vi "transfer char run_subvi_8_24_12a_JW.vi"(0 "VISA session":refnum<visa-resource-name>="GPIB0::17::INSTR", 5 "Var1 sweep settings":T7={"start"=40.0, "stop"=-40.0, "step (linear only)"=-1.0, "sweep spacing (linear: 0)"=0, "sweep mode"=FALSE, "compliance (V)"=100.0, "compliance (A)"=0.001} {"compliance (A)" format="%^.2e"; "compliance (V)" format="%.2f"; "sweep spacing (linear: 0)" items=["linear", "log 10", "log 25", "log 50"]; "step (linear only)" format="%.2f"; "stop" format="%.2f"; "start" format="%.2f"}, 7 "Var2 step settings":T6={"compliance (A)"=0.001, "compliance (V)"=100.0, "start"=-2.0, "total points"=2, "step"=-38.0} {"step" format="%.2f"; "start" format="%.2f"; "compliance (V)" format="%.2f"; "compliance (A)" format="%^.2e"}, 9 "integration time":u32(slide) scale=0.0..2.0, 11 "Input Path":path, 13 "Sample Properties:":T4 {"Date Created" format="%<%x>T"}) -> (2 "Check Cluster":T2, 4 "Output":T3 {"Mobility-Lin" format="%#_4e"; "Mobility-Sat" format="%#_4e"}, 6 "Graph Cluster":T1, 15 "error?":errorcluster)   [LabVIEW 2012]
uses:
  <vilib>/Utility/file.llb/Write To Spreadsheet File (DBL).vi
panel:
  in  "Output Path":path
  in  "Temp (K)":dbl=0.001 format="%^.2e"
  in  "NumPts":dbl=5.0
  out "Numeric":dbl
  out "min r":dbl
  out "max r":dbl
  out "error? 2":errorcluster
  in  "MAXIMUM":ext format="%.2e"
  in  "MINIMUM":ext=-1e-05 format="%_2e"
  out "Gate Current Plot":cluster{"trace":dbl[], "trace":dbl[]}(graph)
  in  "Y1 axis":string="Id"
  in  "Y2 axis settings":T5 {"MAXIMUM" format="%.9f"; "MINIMUM" format="%.9f"}
  out "graphic display":cluster{"trace":dbl[], "trace":dbl[]}(graph)
  in  "wait time parameter":dbl=1.0
  in  "Value (Either V or A) 4":dbl
  in  "Value (Either V or A) 3":dbl
  in  "Value (Either V or A) 2":dbl
  in  "Value (V or A)":dbl
  in  "compliance (A)":dbl=0.001 format="%^.2e"
  in  "compliance (V)":dbl=100.0 format="%^.2e"
  in  "Iname":string="Is"
  in  "Vname":string="Vs"
  in  "Function":u16(ring)=4 items=["disabled", "Var1", "Var2", "Var1'", "Constant"]
  in  "Mode":u16(ring)=4 items=["V", "I", "VPulse", "IPulse", "Common"]
  in  "Iname 4":string="I4"
  in  "Vname 4":string="V4"
  in  "Function 4":u16(ring)=4 items=["disabled", "Var1", "Var2", "Var1'", "Constant"]
  in  "Mode 4":u16(ring) items=["V", "I", "VPulse", "IPulse", "Common"]
  in  "Iname 3":string="Ig"
  in  "Vname 3":string="Vg"
  in  "Function 3":u16(ring)=1 items=["disabled", "Var1", "Var2", "Var1'", "Constant"]
  in  "Mode 3":u16(ring) items=["V", "I", "VPulse", "IPulse", "Common"]
  in  "Iname 2":string="Id"
  in  "Vname 2":string="Vd"
  in  "Function 2":u16(ring)=2 items=["disabled", "Var1", "Var2", "Var1'", "Constant"]
  in  "Mode 2":u16(ring) items=["V", "I", "VPulse", "IPulse", "Common"]
  in  "reset":bool=TRUE
  # "SMU1"
  # "SMU2"
  # "SMU3"
  # "SMU4"
  # "Sample Properties:"
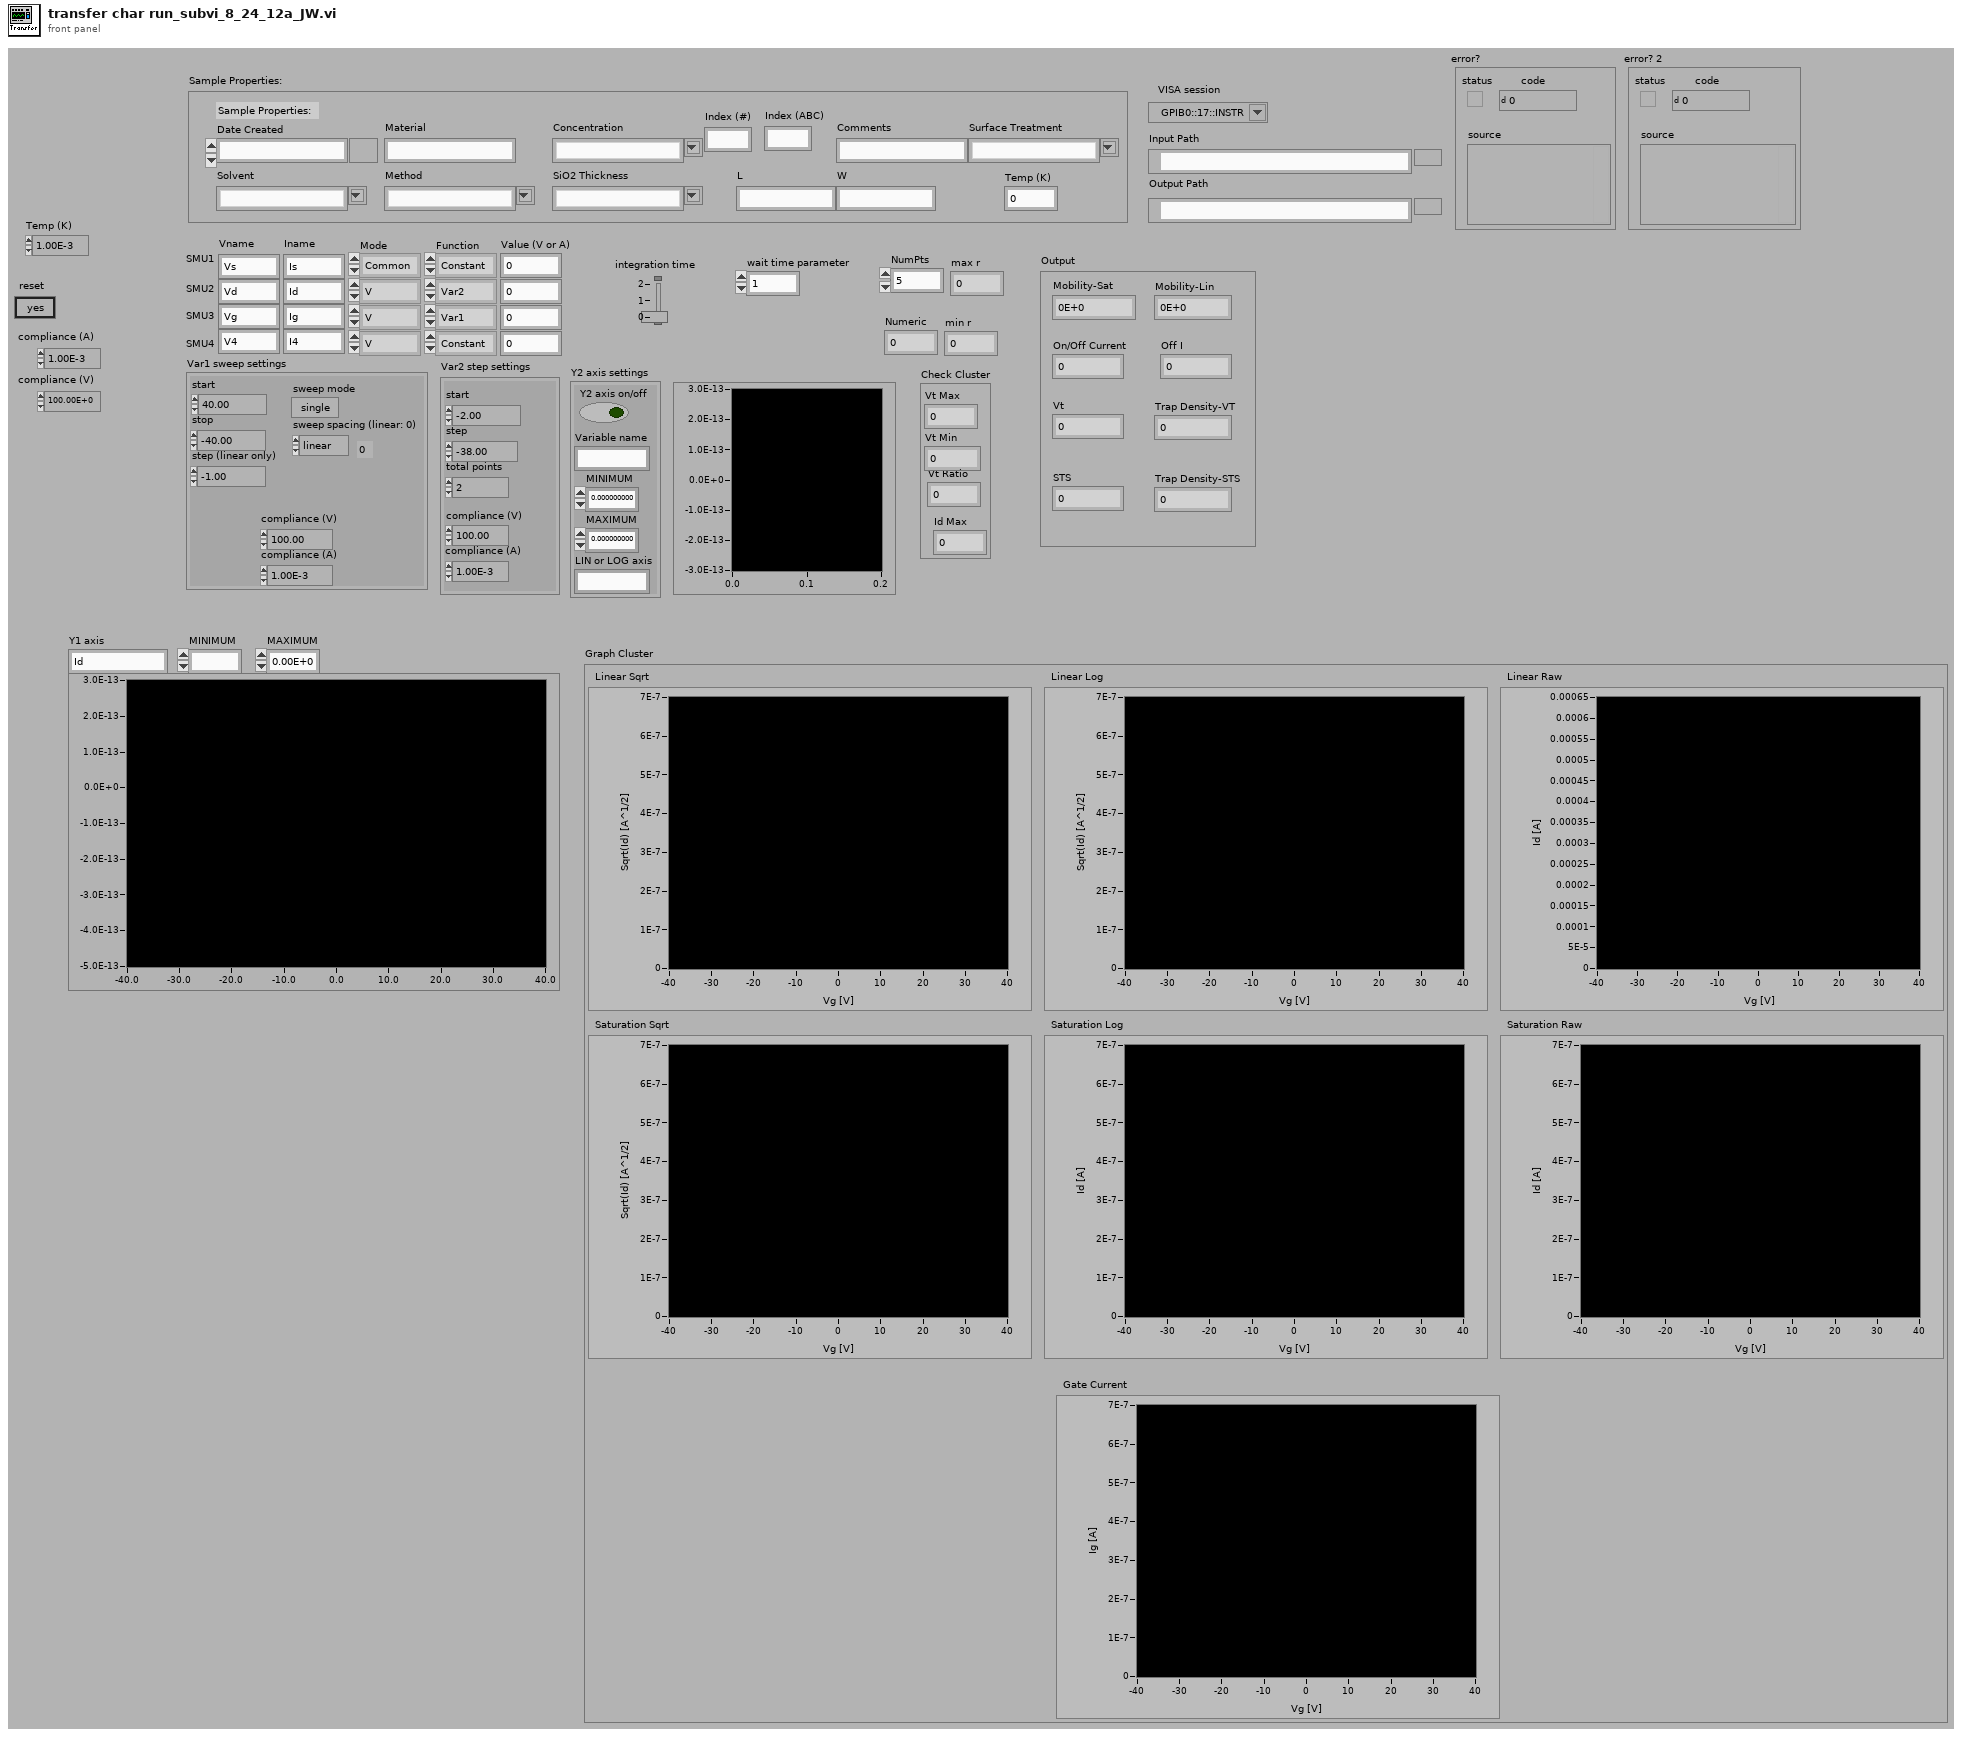
[diagram p1: front panel]
types:
  T1 = cluster{"Linear Sqrt":cluster{dbl[], "trace":dbl[]}[], "Linear Log":cluster{dbl[], "trace":dbl[]}[], "Linear Raw":cluster{dbl[], dbl[]}[], "Saturation Sqrt":cluster{dbl[], "trace":dbl[]}[], "Saturation Log":cluster{dbl[], "trace":dbl[]}[], "Saturation Raw":cluster{dbl[], "trace":dbl[]}[], "Gate Current":cluster{dbl[], "trace":dbl[]}[]}
  T2 = cluster{"Vt Max":i32, "Vt Min":i32, "Vt Ratio":i32, "Id Max":dbl}
  T3 = cluster{"Mobility-Sat":dbl, "Mobility-Lin":dbl, "On/Off Current":dbl, "Off I":dbl, "Vt":dbl, "STS":dbl, "Trap Density-VT":dbl, "Trap Density-STS":dbl}
  T4 = cluster{"Date Created":timestamp, "Material":string, "Solvent":string, "Concentration":string, "Method":string, "SiO2 Thickness":string, "Index (#)":string, "Index (ABC)":string, "L":string, "W":string, "Surface Treatment":string, "Comments":string, "Temp (K)":dbl}
  T5 = cluster{"Y2 axis on/off":bool, "MINIMUM":ext, "MAXIMUM":ext, "Variable name":string, "LIN or LOG axis":string}
  T6 = cluster{"compliance (A)":dbl, "compliance (V)":dbl, "start":dbl, "total points":u16, "step":dbl}
  T7 = cluster{"start":dbl, "stop":dbl, "step (linear only)":dbl, "sweep spacing (linear: 0)":u16, "sweep mode":bool, "compliance (V)":dbl, "compliance (A)":dbl}
  T8 = cluster{"Vt Max":dbl, "Vt Min":dbl, "Vt Ratio":dbl, "Id Max":dbl}
  T9 = cluster{"Mobility-Sat":dbl, "Mobility-Lin":dbl, "On/Off I-Sat":dbl, "Off I-Sat":dbl, "VT-Sat":dbl, "Sub Threshold Swing":dbl, "Trap Density-VT":dbl, "Trap Density (N)":dbl}
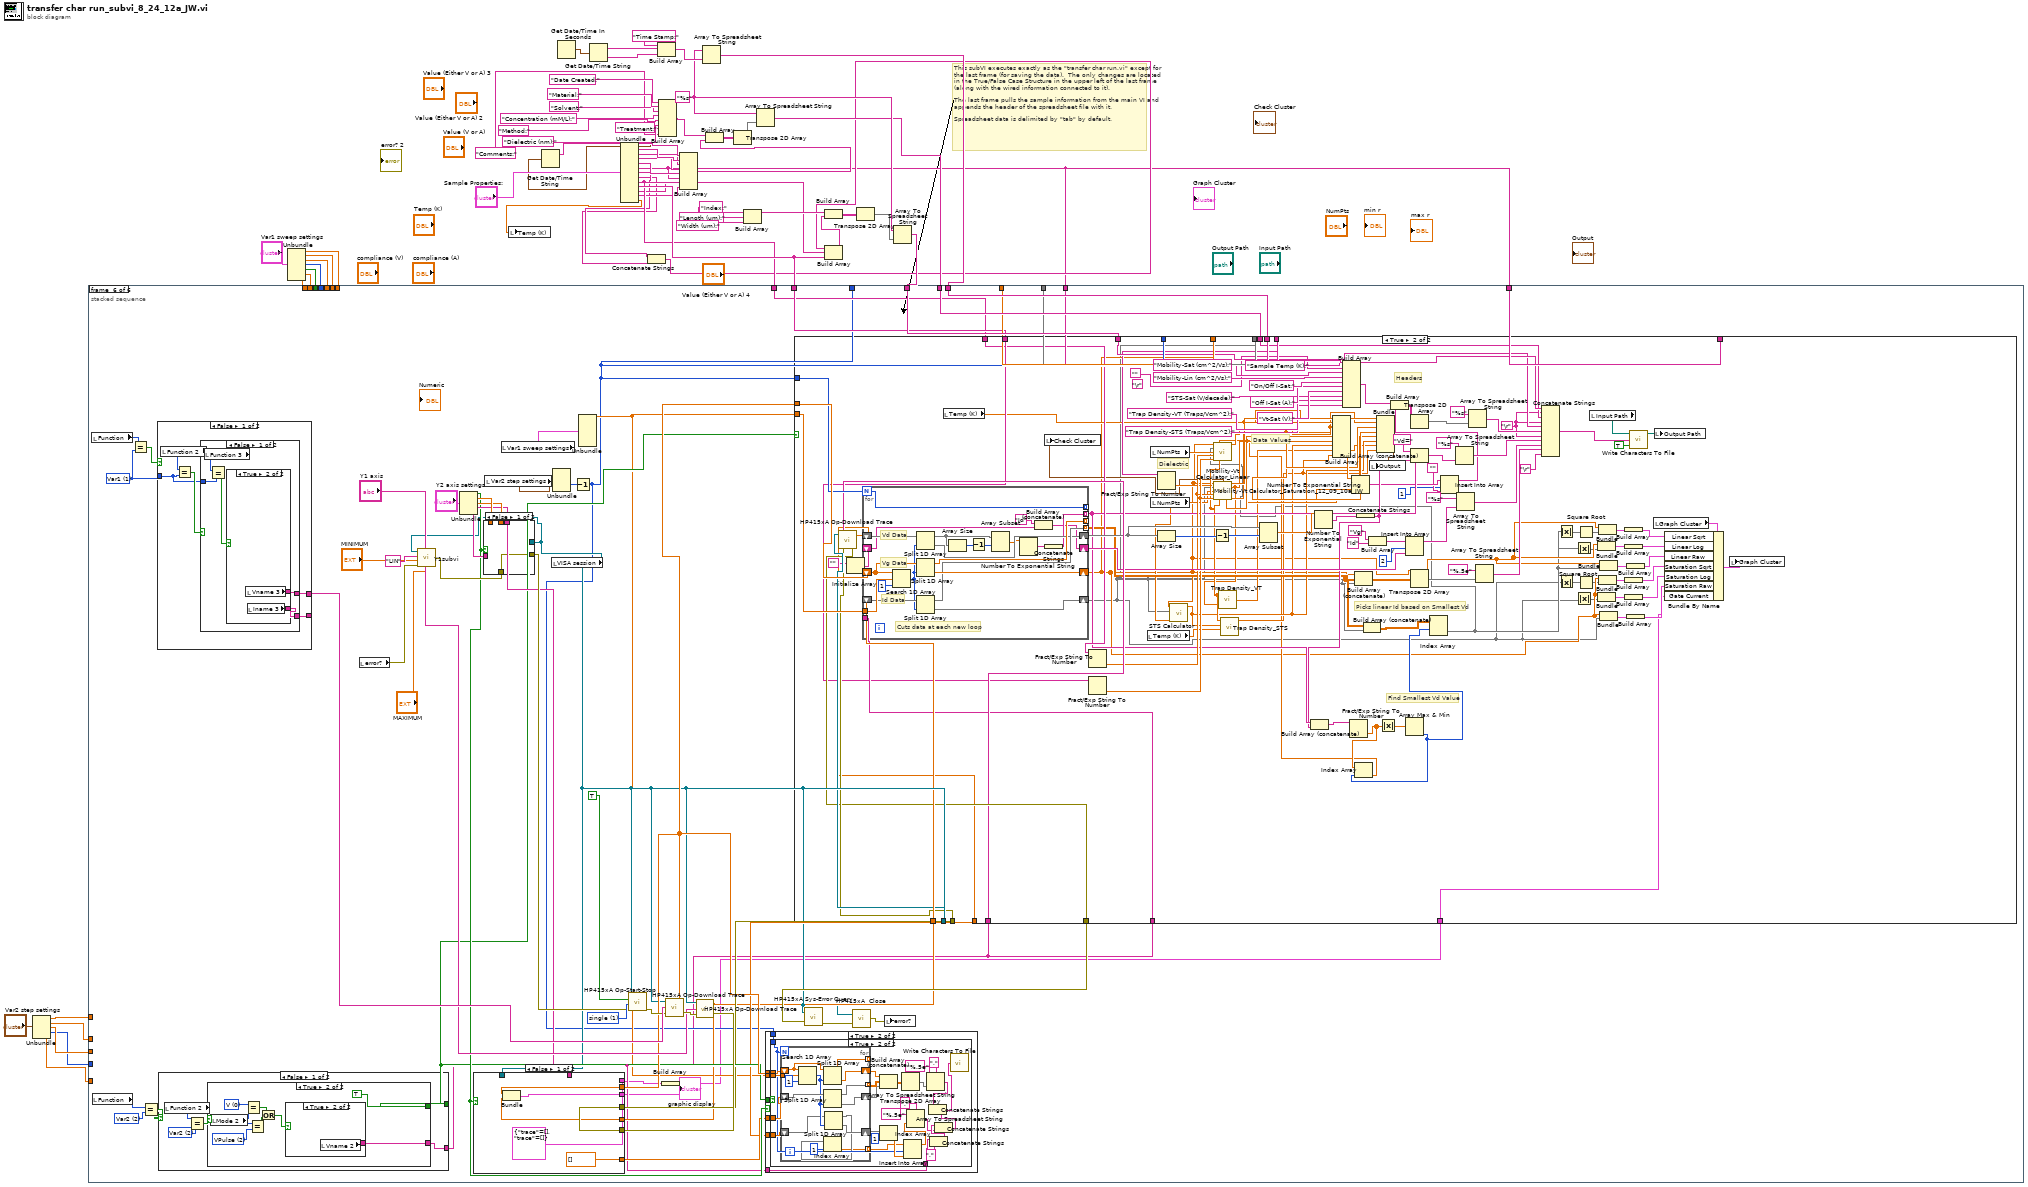
[diagram p0: block diagram]
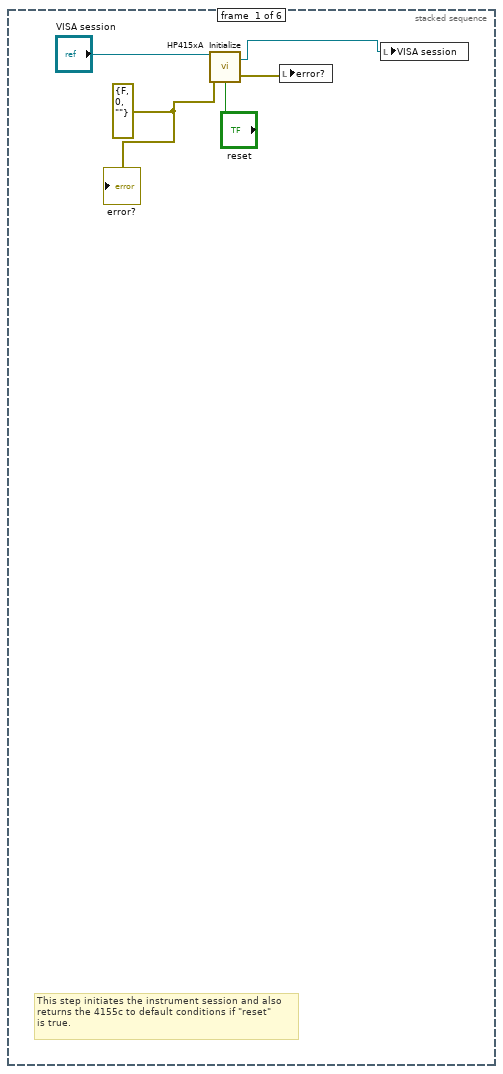
[diagram p2: hidden frame]
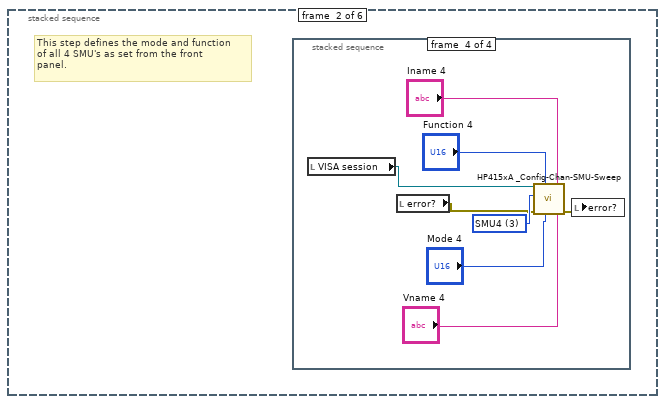
[diagram p3: hidden frame]
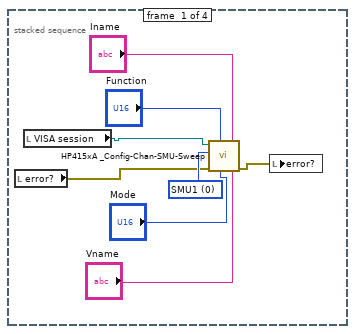
[diagram p4: hidden frame]
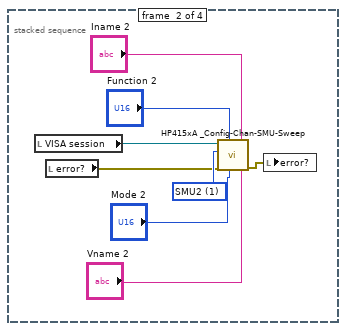
[diagram p5: hidden frame]
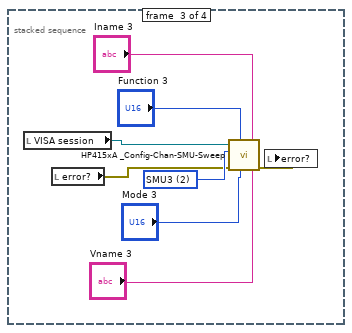
[diagram p6: hidden frame]
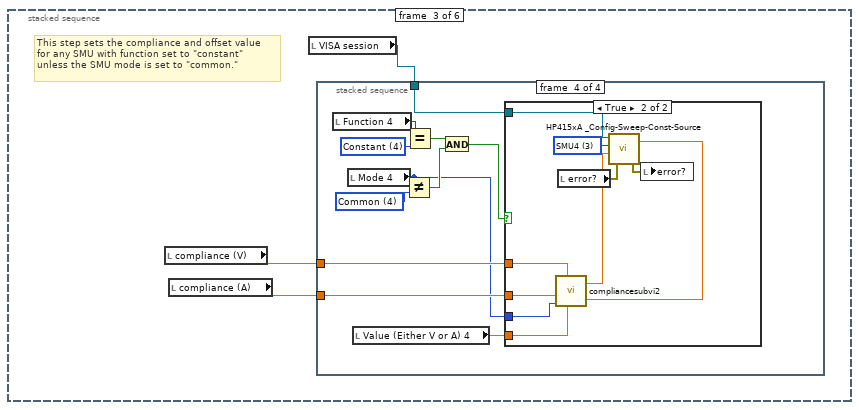
[diagram p7: hidden frame]
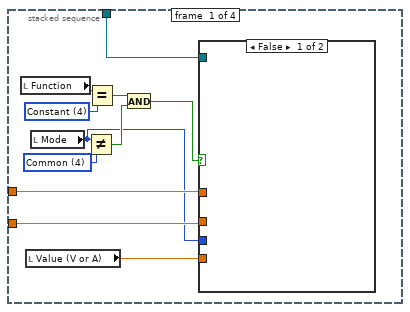
[diagram p8: hidden frame]
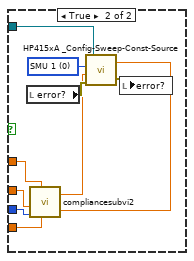
[diagram p9: hidden frame]
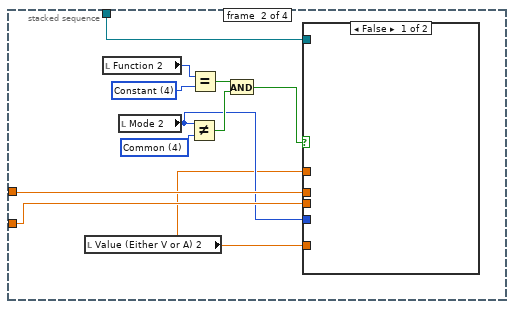
[diagram p10: hidden frame]
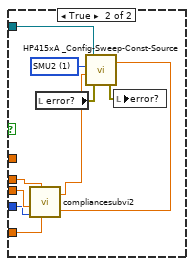
[diagram p11: hidden frame]
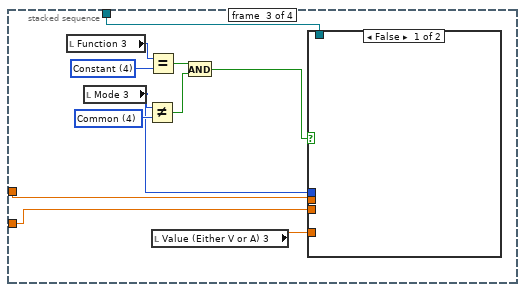
[diagram p12: hidden frame]
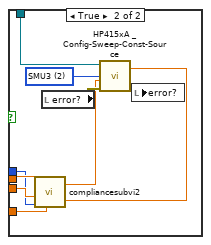
[diagram p13: hidden frame]
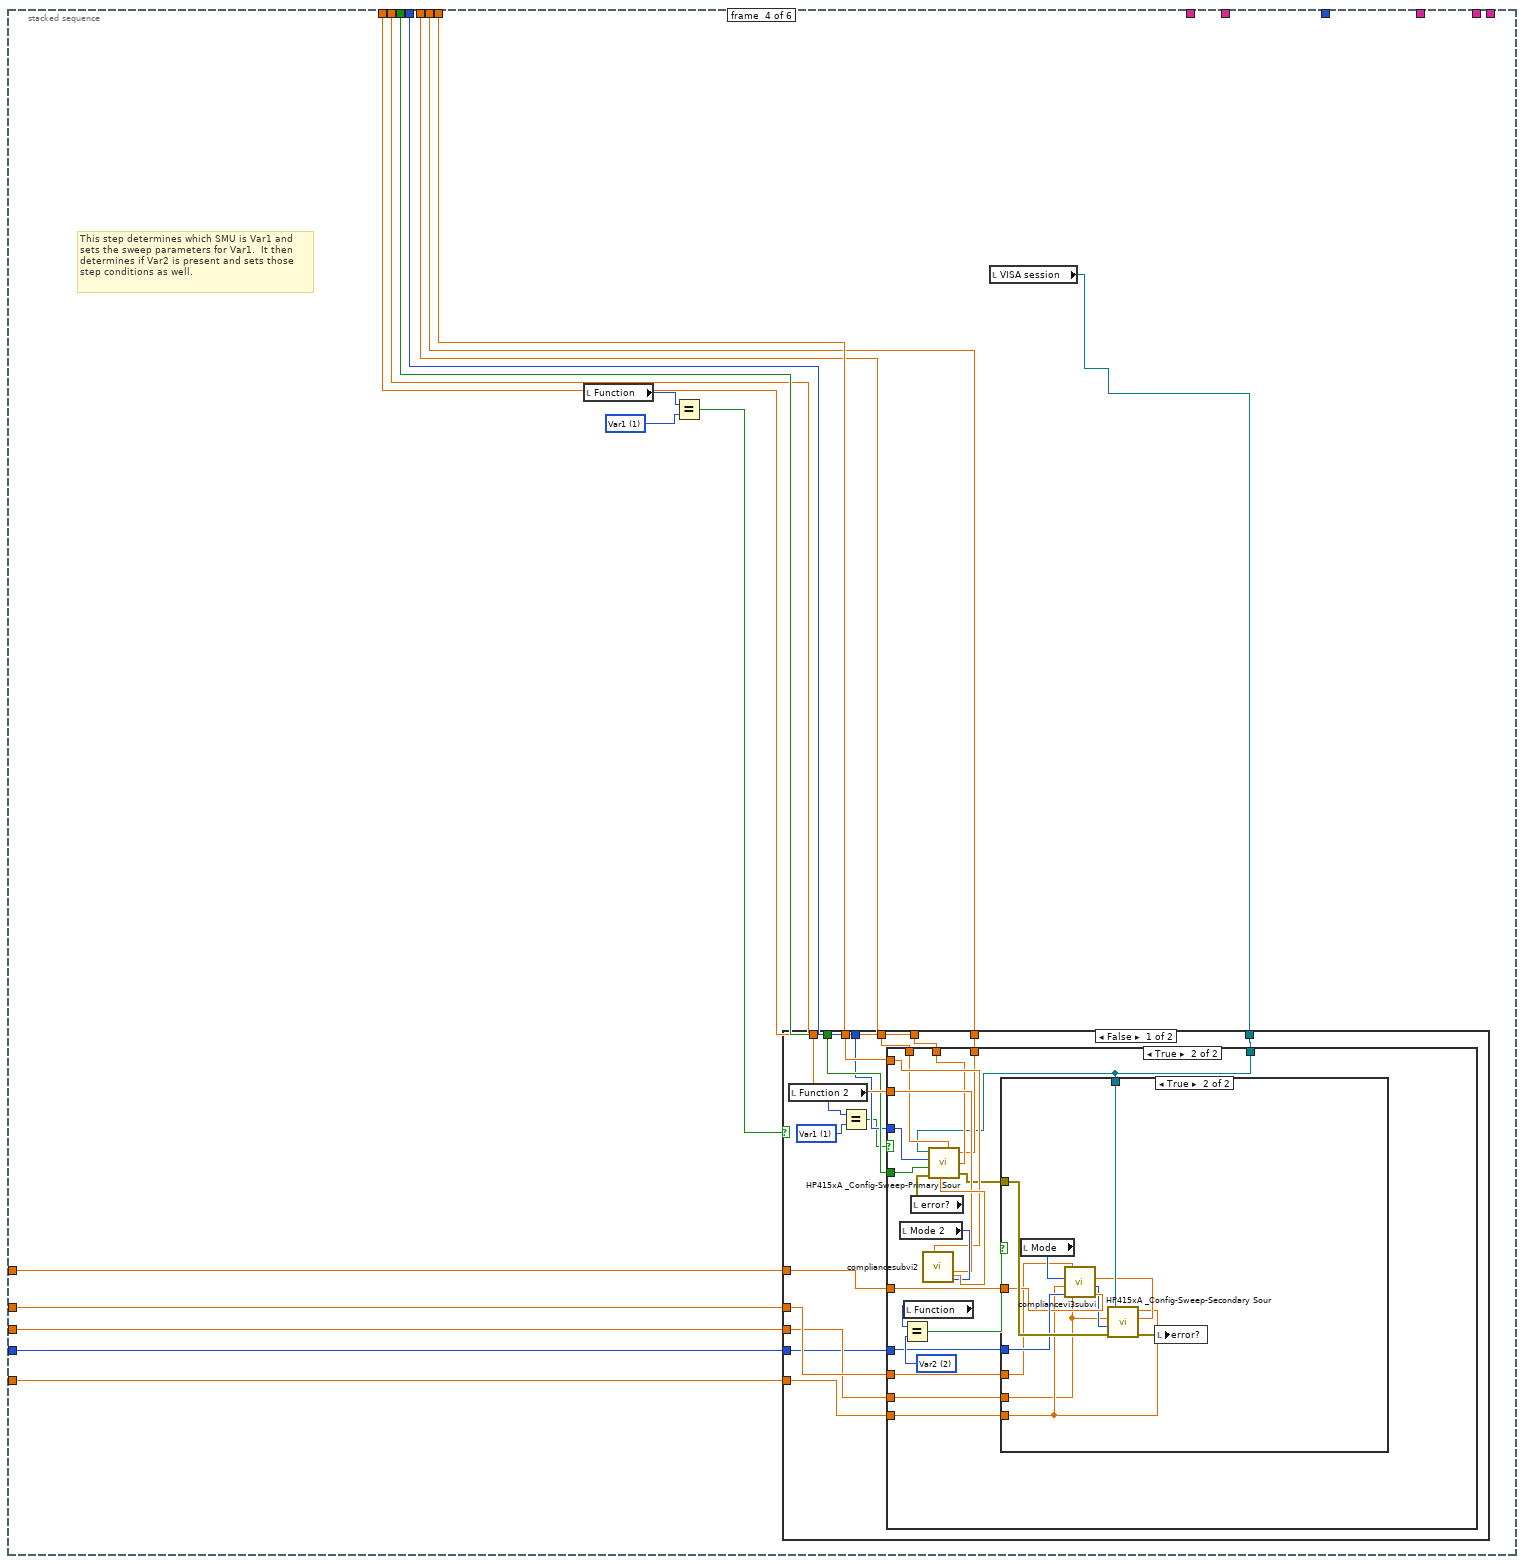
[diagram p15: hidden frame]
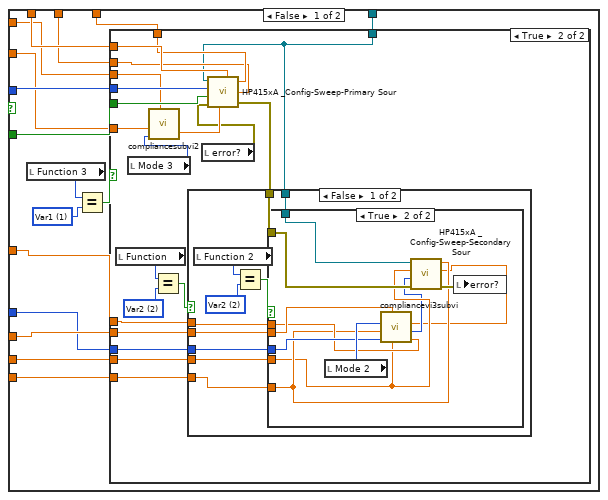
[diagram p16: hidden frame]
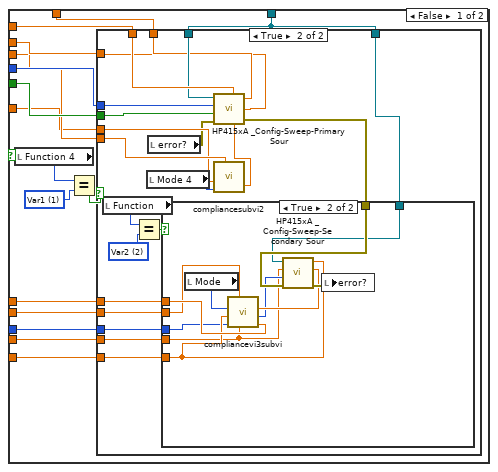
[diagram p17: hidden frame]
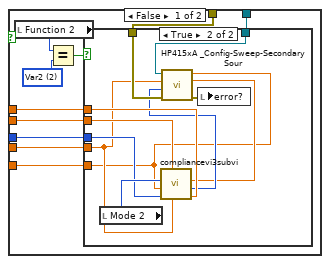
[diagram p19: hidden frame]
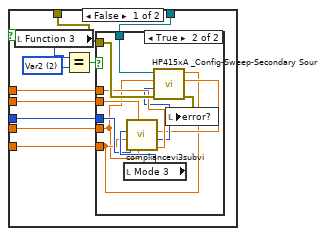
[diagram p20: hidden frame]
diagram:
  w31 = "%s"
  # "This subVI executes exactly as the \"transfer char run.vi\" except for the last frame (for saving the data).  The only changes are located in the True/False Case Structure in the upper left of the last frame (along with the wired information connected to it). \n\nThe last frame pulls the sample information from the main VI and appends the header of the spreadsheet file with it.\n\nSpreadsheet data is delimited by \"tab\" by default."
  n1 = Unbundle("Var2 step settings") -> ("compliance (A)"=w49:dbl, "compliance (V)"=w48:dbl, "start"=w47:dbl, "total points"=w46:u16, "step"=w45:dbl)
  n2 = Unbundle("Var1 sweep settings") -> ("start"=w57:dbl, "stop"=w56:dbl, "step (linear only)"=w55:dbl, "sweep spacing (linear: 0)"=w54:u16, "sweep mode"=w53:bool, "compliance (V)"=w52:dbl, "compliance (A)"=w51:dbl)
  n3 = Get Date/Time In Seconds() -> (seconds since 1Jan1904=w38:timestamp)
  n4 = Get Date/Time String(seconds (now)=w38) -> (date string=w37:string, time string=w36:string)  [unwired: 2 in]
  n5 = Unbundle("Sample Properties:") -> ("Date Created"=w16:timestamp, "Material"=w15:string, "Solvent"=w11:string, "Concentration"=w10:string, "Method"=w14:string, "SiO2 Thickness"=w1:string, "Index (#)"=w5:string, "Index (ABC)"=w4:string, "L"=w8:string, "W"=w9:string, "Surface Treatment"=w7:string, "Comments"=w6:string, "Temp (K)"=w2:dbl)
  n6 = local write "Temp (K)"(w2) -> ()
  n7 = Get Date/Time String(seconds (now)=w16) -> (date string=w43:string)  [unwired: 2 in, 1 out]
  n8 = Concatenate Strings(w5, w4) -> (w3:string)
  n9 = Build Array("Time Stamp:", w37, w36) -> (w35:string[])
  n10 = Build Array("Date Created:", "Material:", "Solvent:", "Concentration (mM/L):", "Method:", "Dielectric (nm):", "Treatment:", "Comments:") -> (w26:string[])
  n11 = Build Array(w43, w15, w11, w10, w14, w1, w7, w6) -> (w25:string[])
  n12 = Array To Spreadsheet String(array=w35, 3:w31) -> (spreadsheet string=w27:string)  [unwired: 1 in]
  n13 = Build Array(w26, w25) -> (w24:string[][])
  n14 = Transpose 2D Array(2D array=w24) -> (transposed array=w23:string[][])
  n15 = Build Array("Index:", "Length (um):", "Width (um):") -> (w22:string[])
  n16 = Array To Spreadsheet String(array=w23, 3:w31) -> (spreadsheet string=w30:string)  [unwired: 1 in]
  n17 = Build Array(w3, w8, w9) -> (w21:string[])
  n18 = Build Array(w22, w21) -> (w20:string[][])
  n19 = Transpose 2D Array(2D array=w20) -> (transposed array=w19:string[][])
  n20 = Array To Spreadsheet String(array=w19, 3:w31) -> (spreadsheet string=w18:string)  [unwired: 1 in]
  n21 = stacked-sequence {
    tunnel: w57 -> [_ _ _ w194 _ _]
    tunnel: w56 -> [_ _ _ w193 _ _]
    tunnel: w55 -> [_ _ _ w192 _ _]
    tunnel: w54 -> [_ _ _ w191 _ _]
    tunnel: w53 -> [_ _ _ w190 _ _]
    tunnel: w52 -> [_ _ _ w189 _ _]
    tunnel: w51 -> [_ _ _ w188 _ _]
    tunnel: w49 -> [_ _ _ w187 _ _]
    tunnel: w48 -> [_ _ _ w186 _ _]
    tunnel: w47 -> [_ _ _ w185 _ _]
    tunnel: w46 -> [_ _ _ w184 _ _]
    tunnel: w45 -> [_ _ _ w183 _ _]
    tunnel: w27 -> [_ _ _ _ _ w562]
    tunnel: w30 -> [_ _ _ _ _ w561]
    tunnel: w18 -> [_ _ _ _ _ w560]
    tunnel: [_ _ _ _ _ w559] -> _
    tunnel: [_ _ _ _ _ w558] -> _
    tunnel: [_ _ _ _ _ w555] -> _
    tunnel: w9 -> [_ _ _ _ _ w557]
    tunnel: w8 -> [_ _ _ _ _ w556]
    tunnel: w1 -> [_ _ _ _ _ w554]
    tunnel: w1 -> [_ _ _ _ _ w553]
    frame #0 {
      w62 = errorcluster {"status"=FALSE, "code"=0, "source"=""} ("error out")
      # "This step initiates the instrument session and also\nreturns the 4155c to default conditions if \"reset\"\nis true."
      n22 = call "HP415xA  Initialize.vi"("instrument descriptor"="VISA session", "reset"="reset", "error in (no error)"=w62) -> ("VISA session"=w59:refnum<visa-resource-name>, "error out"=w61:errorcluster)  [unwired: 2 in]
      n23 = local write "error?"(w61) -> ()
      n24 = local write "VISA session"(w59) -> ()
      "error?" <- w62
    }
    frame #1 {
      # "This step defines the mode and function\nof all 4 SMU's as set from the front\npanel."
      n25 = stacked-sequence {
        frame #0 {
          w71 = u32 0 items=["SMU1  ", "SMU2  ", "SMU3  ", "SMU4  ", "SMU5  ", "SMU6  "] ("unit to configure")
          n26 = local read "error?"() -> (w66:errorcluster)
          n27 = local read "VISA session"() -> (w64:refnum<visa-resource-name>)
          n28 = call "HP415xA _Config-Chan-SMU-Sweep.vi"("V name (max 6 chars)"="Vname", "I name (max 6 chars)"="Iname", "mode"="Mode", "function"="Function", "error in (no error)"=w66, "unit to configure"=w71, "VISA session"=w64) -> ("error out"=w65:errorcluster)  [unwired: 2 in]
          n29 = local write "error?"(w65) -> ()
        }
        frame #1 {
          w75 = u32 1 items=["SMU1  ", "SMU2  ", "SMU3  ", "SMU4  ", "SMU5  ", "SMU6  "] ("unit to configure")
          n30 = local read "VISA session"() -> (w72:refnum<visa-resource-name>)
          n31 = local read "error?"() -> (w73:errorcluster)
          n32 = call "HP415xA _Config-Chan-SMU-Sweep.vi"("V name (max 6 chars)"="Vname 2", "I name (max 6 chars)"="Iname 2", "mode"="Mode 2", "function"="Function 2", "error in (no error)"=w73, "unit to configure"=w75, "VISA session"=w72) -> ("error out"=w74:errorcluster)  [unwired: 2 in]
          n33 = local write "error?"(w74) -> ()
        }
        frame #2 {
          w83 = u32 2 items=["SMU1  ", "SMU2  ", "SMU3  ", "SMU4  ", "SMU5  ", "SMU6  "] ("unit to configure")
          n34 = local read "VISA session"() -> (w80:refnum<visa-resource-name>)
          n35 = local read "error?"() -> (w81:errorcluster)
          n36 = call "HP415xA _Config-Chan-SMU-Sweep.vi"("V name (max 6 chars)"="Vname 3", "I name (max 6 chars)"="Iname 3", "mode"="Mode 3", "function"="Function 3", "error in (no error)"=w81, "unit to configure"=w83, "VISA session"=w80) -> ("error out"=w82:errorcluster)  [unwired: 2 in]
          n37 = local write "error?"(w82) -> ()
        }
        frame #3 {
          w91 = u32 3 items=["SMU1  ", "SMU2  ", "SMU3  ", "SMU4  ", "SMU5  ", "SMU6  "] ("unit to configure")
          n38 = local read "VISA session"() -> (w88:refnum<visa-resource-name>)
          n39 = local read "error?"() -> (w90:errorcluster)
          n40 = call "HP415xA _Config-Chan-SMU-Sweep.vi"("V name (max 6 chars)"="Vname 4", "I name (max 6 chars)"="Iname 4", "mode"="Mode 4", "function"="Function 4", "error in (no error)"=w90, "unit to configure"=w91, "VISA session"=w88) -> ("error out"=w89:errorcluster)  [unwired: 2 in]
          n41 = local write "error?"(w89) -> ()
        }
      }
    }
    frame #2 {
      # "This step sets the compliance and offset value\nfor any SMU with function set to \"constant\"\nunless the SMU mode is set to \"common.\""
      n42 = local read "compliance (V)"() -> (w97:dbl)
      n43 = local read "compliance (A)"() -> (w98:dbl)
      n44 = local read "VISA session"() -> (w96:refnum<visa-resource-name>)
      n45 = stacked-sequence {
        tunnel: w96 -> [w107 w127 w146 w166]
        tunnel: w98 -> [w101 w123 w144 w164]
        tunnel: w97 -> [w100 w122 w143 w165]
        frame #0 {
          w105 = u16 4 items=["V", "I", "VPulse", "IPulse", "Common"] ("Mode")
          w109 = u16 4 items=["disabled", "Var1", "Var2", "Var1'", "Constant"] ("Function")
          n46 = local read "Function"() -> (w108:u16)
          n47 = local read "Value (V or A)"() -> (w102:dbl)
          n48 = local read "Mode"() -> (w99:u16)
          n49 = Not Equal?(x=w99, y=w105) -> (x != y?=w104:bool)
          n50 = Equal?(x=w108, y=w109) -> (x = y?=w106:bool)
          n51 = And(x=w106, y=w104) -> (x .and. y?=w103:bool)
          n52 = case shown="False" w103 {
            tunnel: w107 -> [_ w119]
            tunnel: w100 -> [_ w115]
            tunnel: w101 -> [_ w114]
            tunnel: w102 -> [_ w111]
            tunnel: w99 -> [_ w112]
            frame False {
            }
            frame True {
              w118 = u16 0 items=["SMU 1", "SMU2", "SMU3", "SMU4", "SMU5", "SMU6", "VSU1", "VSU2"] ("unit (SMU1:0)")
              n53 = local read "error?"() -> (w117:errorcluster)
              n54 = call "compliancesubvi2.vi"("Value1"=w111, "compliance (V)"=w115, "Mode"=w112, "compliance (A)"=w114) -> ("compliance"=w113:dbl, "constant"=w110:dbl)  [unwired: 2 in]
              n55 = call "HP415xA _Config-Sweep-Const-Source.vi"("compliance (SMUs only)"=w113, "error in (no error)"=w117, "source (V or A)"=w110, "unit (SMU1:0)"=w118, "VISA session"=w119) -> ("error out"=w116:errorcluster)
              n56 = local write "error?"(w116) -> ()
            }
          }
        }
        frame #1 {
          w124 = u16 4 items=["V", "I", "VPulse", "IPulse", "Common"] ("Mode 2")
          w125 = u16 4 items=["disabled", "Var1", "Var2", "Var1'", "Constant"] ("Function 2")
          n57 = local read "Value (Either V or A) 2"() -> (w120:dbl)
          n58 = local read "Function 2"() -> (w126:u16)
          n59 = local read "Mode 2"() -> (w121:u16)
          n60 = Not Equal?(x=w121, y=w124) -> (x != y?=w129:bool)
          n61 = Equal?(x=w126, y=w125) -> (x = y?=w130:bool)
          n62 = And(x=w130, y=w129) -> (x .and. y?=w128:bool)
          n63 = case shown="False" w128 {
            tunnel: w127 -> [_ w140]
            tunnel: w122 -> [_ w138]
            tunnel: w123 -> [_ w137]
            tunnel: w120 -> [_ _]
            tunnel: w121 -> [_ w133]
            tunnel: w120 -> [_ w132]
            frame False {
            }
            frame True {
              w139 = u16 1 items=["SMU 1", "SMU2", "SMU3", "SMU4", "SMU5", "SMU6", "VSU1", "VSU2"] ("unit (SMU1:0)")
              n64 = call "compliancesubvi2.vi"("Value1"=w132, "compliance (V)"=w138, "Mode"=w133, "compliance (A)"=w137) -> ("compliance"=w136:dbl, "constant"=w131:dbl)  [unwired: 2 in]
              n65 = local read "error?"() -> (w135:errorcluster)
              n66 = call "HP415xA _Config-Sweep-Const-Source.vi"("compliance (SMUs only)"=w136, "error in (no error)"=w135, "source (V or A)"=w131, "unit (SMU1:0)"=w139, "VISA session"=w140) -> ("error out"=w134:errorcluster)
              n67 = local write "error?"(w134) -> ()
            }
          }
        }
        frame #2 {
          w148 = u16 4 items=["V", "I", "VPulse", "IPulse", "Common"] ("Mode 2")
          w149 = u16 4 items=["disabled", "Var1", "Var2", "Var1'", "Constant"] ("Function 2")
          n68 = local read "Function 3"() -> (w147:u16)
          n69 = local read "Mode 3"() -> (w142:u16)
          n70 = Not Equal?(x=w142, y=w148) -> (x != y?=w150:bool)
          n71 = Equal?(x=w147, y=w149) -> (x = y?=w151:bool)
          n72 = local read "Value (Either V or A) 3"() -> (w145:dbl)
          n73 = And(x=w151, y=w150) -> (x .and. y?=w141:bool)
          n74 = case shown="False" w141 {
            tunnel: w146 -> [_ w159]
            tunnel: w145 -> [_ w153]
            tunnel: w144 -> [_ w156]
            tunnel: w143 -> [_ w155]
            tunnel: w142 -> [_ w154]
            frame False {
            }
            frame True {
              w158 = u16 2 items=["SMU 1", "SMU2", "SMU3", "SMU4", "SMU5", "SMU6", "VSU1", "VSU2"] ("unit (SMU1:0)")
              n75 = call "compliancesubvi2.vi"("Value1"=w153, "compliance (V)"=w155, "Mode"=w154, "compliance (A)"=w156) -> ("compliance"=w157:dbl, "constant"=w152:dbl)  [unwired: 2 in]
              n76 = local read "error?"() -> (w161:errorcluster)
              n77 = call "HP415xA _Config-Sweep-Const-Source.vi"("compliance (SMUs only)"=w157, "error in (no error)"=w161, "source (V or A)"=w152, "unit (SMU1:0)"=w158, "VISA session"=w159) -> ("error out"=w160:errorcluster)
              n78 = local write "error?"(w160) -> ()
            }
          }
        }
        frame #3 {
          w168 = u16 4 items=["V", "I", "VPulse", "IPulse", "Common"] ("Mode 4")
          w169 = u16 4 items=["disabled", "Var1", "Var2", "Var1'", "Constant"] ("Function 4")
          n79 = local read "Function 4"() -> (w170:u16)
          n80 = local read "Mode 4"() -> (w163:u16)
          n81 = local read "Value (Either V or A) 4"() -> (w162:dbl)
          n82 = Not Equal?(x=w163, y=w168) -> (x != y?=w171:bool)
          n83 = Equal?(x=w170, y=w169) -> (x = y?=w172:bool)
          n84 = And(x=w172, y=w171) -> (x .and. y?=w167:bool)
          n85 = case shown="True" w167 {
            tunnel: w166 -> [_ w181]
            tunnel: w165 -> [_ w177]
            tunnel: w164 -> [_ w178]
            tunnel: w163 -> [_ w176]
            tunnel: w162 -> [_ w175]
            frame False {
            }
            frame True {
              w182 = u16 3 items=["SMU 1", "SMU2", "SMU3", "SMU4", "SMU5", "SMU6", "VSU1", "VSU2"] ("unit (SMU1:0)")
              n86 = call "compliancesubvi2.vi"("Value1"=w175, "compliance (V)"=w177, "Mode"=w176, "compliance (A)"=w178) -> ("compliance"=w174:dbl, "constant"=w173:dbl)  [unwired: 2 in]
              n87 = local read "error?"() -> (w180:errorcluster)
              n88 = call "HP415xA _Config-Sweep-Const-Source.vi"("compliance (SMUs only)"=w174, "error in (no error)"=w180, "source (V or A)"=w173, "unit (SMU1:0)"=w182, "VISA session"=w181) -> ("error out"=w179:errorcluster)
              n89 = local write "error?"(w179) -> ()
            }
          }
        }
      }
    }
    frame #3 {
      w198 = u16 1 items=["disabled", "Var1", "Var2", "Var1'", "Constant"] ("Function")
      # "This step determines which SMU is Var1 and\nsets the sweep parameters for Var1.  It then\ndetermines if Var2 is present and sets those\nstep conditions as well."
      n90 = local read "Function"() -> (w197:u16)
      n91 = Equal?(x=w197, y=w198) -> (x = y?=w196:bool)
      n92 = local read "VISA session"() -> (w195:refnum<visa-resource-name>)
      n93 = case shown="False" w196 {
        tunnel: w189 -> [w211 w487]
        tunnel: w188 -> [w212 w486]
        tunnel: w191 -> [w209 w485]
        tunnel: w190 -> [w210 w484]
        tunnel: w192 -> [w206 w483]
        tunnel: w193 -> [w205 w482]
        tunnel: w194 -> [w207 w481]
        tunnel: w195 -> [w208 w470]
        tunnel: w187 -> [w203 w476]
        tunnel: w186 -> [w202 w475]
        tunnel: w185 -> [w201 w474]
        tunnel: w184 -> [w200 w473]
        tunnel: w183 -> [w199 w472]
        frame False {
          w214 = u16 1 items=["disabled", "Var1", "Var2", "Var1'", "Constant"] ("Function")
          n94 = local read "Function 2"() -> (w213:u16)
          n95 = Equal?(x=w213, y=w214) -> (x = y?=w204:bool)
          n96 = case shown="True" w204 {
            tunnel: w212 -> [w220 w413]
            tunnel: w211 -> [w221 w412]
            tunnel: w210 -> [w222 w411]
            tunnel: w209 -> [w223 w410]
            tunnel: w208 -> [w227 w399]
            tunnel: w207 -> [w226 w409]
            tunnel: w206 -> [w224 w408]
            tunnel: w205 -> [w225 w407]
            tunnel: w203 -> [w219 w402]
            tunnel: w202 -> [w218 w401]
            tunnel: w201 -> [w216 w400]
            tunnel: w200 -> [w217 w397]
            tunnel: w199 -> [w215 w396]
            frame False {
              w230 = u16 1 items=["disabled", "Var1", "Var2", "Var1'", "Constant"] ("Function")
              n97 = local read "Function 3"() -> (w229:u16)
              n98 = Equal?(x=w229, y=w230) -> (x = y?=w228:bool)
              n99 = case shown="True" w228 {
                tunnel: w227 -> [w231 w324]
                tunnel: w226 -> [w243 w341]
                tunnel: w225 -> [w240 w340]
                tunnel: w224 -> [w239 w339]
                tunnel: w223 -> [w242 w338]
                tunnel: w222 -> [w241 w337]
                tunnel: w221 -> [w238 w336]
                tunnel: w220 -> [w237 w335]
                tunnel: w219 -> [w236 w328]
                tunnel: w218 -> [w235 w327]
                tunnel: w217 -> [w234 w326]
                tunnel: w216 -> [w233 w323]
                tunnel: w215 -> [w232 w322]
                frame False {
                  w246 = u16 1 items=["disabled", "Var1", "Var2", "Var1'", "Constant"] ("Function")
                  n100 = local read "Function 4"() -> (w245:u16)
                  n101 = Equal?(x=w245, y=w246) -> (x = y?=w244:bool)
                  n102 = case shown="True" w244 {
                    tunnel: w243 -> [_ w265]
                    tunnel: w231 -> [_ w264]
                    tunnel: w242 -> [_ w263]
                    tunnel: w241 -> [_ w262]
                    tunnel: w240 -> [_ w261]
                    tunnel: w239 -> [_ w260]
                    tunnel: w238 -> [_ w259]
                    tunnel: w237 -> [_ w258]
                    tunnel: w236 -> [_ w253]
                    tunnel: w235 -> [_ w252]
                    tunnel: w234 -> [_ w251]
                    tunnel: w233 -> [_ w250]
                    tunnel: w232 -> [_ w249]
                    tunnel: w231 -> [_ w247]
                    frame False {
                    }
                    frame True {
                      w256 = u16 2 items=["disabled", "Var1", "Var2", "Var1'", "Constant"] ("Function")
                      n103 = local read "Function"() -> (w255:u16)
                      n104 = Equal?(x=w255, y=w256) -> (x = y?=w254:bool)
                      n105 = local read "Mode 4"() -> (w267:u16)
                      n106 = local read "error?"() -> (w257:errorcluster)
                      n107 = call "compliancesubvi2.vi"("compliance (V)"=w259, "Mode"=w267, "compliance (A)"=w258) -> ("compliance"=w266:dbl)  [unwired: 3 in, 1 out]
                      n108 = call "HP415xA _Config-Sweep-Primary Sour.vi"("step (linear only)"=w260, "stop"=w261, "start"=w265, "compliance"=w266, "error in (no error)"=w257, "sweep mode"=w262, "sweep spacing (linear: 0)"=w263, "VISA session"=w264) -> ("error out"=w248:errorcluster)  [unwired: 2 in]
                      n109 = case shown="True" w254 {
                        tunnel: w253 -> [w274 w317]
                        tunnel: w252 -> [w273 w312]
                        tunnel: w251 -> [w272 w311]
                        tunnel: w250 -> [w271 w313]
                        tunnel: w249 -> [w270 w316]
                        tunnel: w248 -> [w269 w319]
                        tunnel: w247 -> [w268 w318]
                        frame False {
                          w277 = u16 2 items=["disabled", "Var1", "Var2", "Var1'", "Constant"] ("Function")
                          n110 = local read "Function 2"() -> (w276:u16)
                          n111 = Equal?(x=w276, y=w277) -> (x = y?=w275:bool)
                          n112 = case shown="True" w275 {
                            tunnel: w274 -> [w285 w305]
                            tunnel: w273 -> [w284 w306]
                            tunnel: w272 -> [w283 w304]
                            tunnel: w271 -> [w282 w302]
                            tunnel: w270 -> [w281 w300]
                            tunnel: w269 -> [w280 w310]
                            tunnel: w268 -> [w278 w309]
                            frame False {
                              w287 = u16 2 items=["disabled", "Var1", "Var2", "Var1'", "Constant"] ("Function")
                              n113 = local read "Function 3"() -> (w279:u16)
                              n114 = Equal?(x=w279, y=w287) -> (x = y?=w286:bool)
                              n115 = case shown="True" w286 {
                                tunnel: w285 -> [_ w293]
                                tunnel: w284 -> [_ w294]
                                tunnel: w283 -> [_ w295]
                                tunnel: w282 -> [_ w289]
                                tunnel: w281 -> [_ w290]
                                tunnel: w280 -> [w288 w299]
                                tunnel: w278 -> [_ w298]
                                frame False {
                                n116 = local write "error?"(w288) -> ()
                                }
                                frame True {
                                n117 = local read "Mode 3"() -> (w297:u16)
                                n118 = call "compliancevi3subvi.vi"("compliance (A)"=w293, "start"=w289, "compliance (V)"=w294, "total points"=w295, "step"=w290, "Mode"=w297) -> ("total points 2"=w292:u16, "compliance"=w291:dbl)  [unwired: 1 in, 1 out]
                                n119 = call "HP415xA _Config-Sweep-Secondary Sour.vi"("compliance"=w291, "step"=w290, "error in (no error)"=w299, "total points"=w292, "start"=w289, "VISA session"=w298) -> ("error out"=w296:errorcluster)  [unwired: 1 in]
                                n120 = local write "error?"(w296) -> ()
                                }
                              }
                            }
                            frame True {
                              n121 = local read "Mode 2"() -> (w308:u16)
                              n122 = call "compliancevi3subvi.vi"("compliance (A)"=w305, "start"=w302, "compliance (V)"=w306, "total points"=w304, "step"=w300, "Mode"=w308) -> ("total points 2"=w303:u16, "compliance"=w301:dbl)  [unwired: 1 in, 1 out]
                              n123 = call "HP415xA _Config-Sweep-Secondary Sour.vi"("compliance"=w301, "step"=w300, "error in (no error)"=w310, "total points"=w303, "start"=w302, "VISA session"=w309) -> ("error out"=w307:errorcluster)  [unwired: 1 in]
                              n124 = local write "error?"(w307) -> ()
                            }
                          }
                        }
                        frame True {
                          n125 = local read "Mode"() -> (w321:u16)
                          n126 = call "compliancevi3subvi.vi"("compliance (A)"=w317, "start"=w313, "compliance (V)"=w312, "total points"=w311, "step"=w316, "Mode"=w321) -> ("total points 2"=w314:u16, "compliance"=w315:dbl)  [unwired: 1 in, 1 out]
                          n127 = call "HP415xA _Config-Sweep-Secondary Sour.vi"("compliance"=w315, "step"=w316, "error in (no error)"=w319, "total points"=w314, "start"=w313, "VISA session"=w318) -> ("error out"=w320:errorcluster)  [unwired: 1 in]
                          n128 = local write "error?"(w320) -> ()
                        }
                      }
                    }
                  }
                }
                frame True {
                  w331 = u16 2 items=["disabled", "Var1", "Var2", "Var1'", "Constant"] ("Function")
                  n129 = local read "Function"() -> (w330:u16)
                  n130 = local read "Mode 3"() -> (w333:u16)
                  n131 = call "compliancesubvi2.vi"("compliance (V)"=w336, "Mode"=w333, "compliance (A)"=w335) -> ("compliance"=w334:dbl)  [unwired: 3 in, 1 out]
                  n132 = Equal?(x=w330, y=w331) -> (x = y?=w329:bool)
                  n133 = local read "error?"() -> (w332:errorcluster)
                  n134 = call "HP415xA _Config-Sweep-Primary Sour.vi"("step (linear only)"=w339, "stop"=w340, "start"=w341, "compliance"=w334, "error in (no error)"=w332, "sweep mode"=w337, "sweep spacing (linear: 0)"=w338, "VISA session"=w324) -> ("error out"=w325:errorcluster)  [unwired: 2 in]
                  n135 = case shown="False" w329 {
                    tunnel: w328 -> [w346 w391]
                    tunnel: w327 -> [w345 w390]
                    tunnel: w326 -> [w343 w389]
                    tunnel: w325 -> [w348 w394]
                    tunnel: w324 -> [w347 w393]
                    tunnel: w323 -> [w342 w386]
                    tunnel: w322 -> [w344 w385]
                    frame False {
                      w351 = u16 2 items=["disabled", "Var1", "Var2", "Var1'", "Constant"] ("Function")
                      n136 = local read "Function 2"() -> (w350:u16)
                      n137 = Equal?(x=w350, y=w351) -> (x = y?=w349:bool)
                      n138 = case shown="True" w349 {
                        tunnel: w348 -> [w358 w383]
                        tunnel: w347 -> [w357 w382]
                        tunnel: w346 -> [w356 w378]
                        tunnel: w345 -> [w355 w379]
                        tunnel: w344 -> [w352 w377]
                        tunnel: w343 -> [w354 w380]
                        tunnel: w342 -> [w353 w376]
                        frame False {
                          w361 = u16 2 items=["disabled", "Var1", "Var2", "Var1'", "Constant"] ("Function")
                          n139 = local read "Function 4"() -> (w360:u16)
                          n140 = Equal?(x=w360, y=w361) -> (x = y?=w359:bool)
                          n141 = case shown="True" w359 {
                            tunnel: w358 -> [w362 w371]
                            tunnel: w357 -> [_ w372]
                            tunnel: w356 -> [_ w368]
                            tunnel: w355 -> [_ w369]
                            tunnel: w354 -> [_ w367]
                            tunnel: w353 -> [_ w364]
                            tunnel: w352 -> [_ w363]
                            frame False {
                              n142 = local write "error?"(w362) -> ()
                            }
                            frame True {
                              n143 = local read "Mode 4"() -> (w373:u16)
                              n144 = call "compliancevi3subvi.vi"("compliance (A)"=w368, "start"=w364, "compliance (V)"=w369, "total points"=w367, "step"=w363, "Mode"=w373) -> ("total points 2"=w366:u16, "compliance"=w365:dbl)  [unwired: 1 in, 1 out]
                              n145 = call "HP415xA _Config-Sweep-Secondary Sour.vi"("compliance"=w365, "step"=w363, "error in (no error)"=w371, "total points"=w366, "start"=w364, "VISA session"=w372) -> ("error out"=w370:errorcluster)  [unwired: 1 in]
                              n146 = local write "error?"(w370) -> ()
                            }
                          }
                        }
                        frame True {
                          n147 = local read "Mode 2"() -> (w384:u16)
                          n148 = call "compliancevi3subvi.vi"("compliance (A)"=w378, "start"=w376, "compliance (V)"=w379, "total points"=w380, "step"=w377, "Mode"=w384) -> ("total points 2"=w375:u16, "compliance"=w374:dbl)  [unwired: 1 in, 1 out]
                          n149 = call "HP415xA _Config-Sweep-Secondary Sour.vi"("compliance"=w374, "step"=w377, "error in (no error)"=w383, "total points"=w375, "start"=w376, "VISA session"=w382) -> ("error out"=w381:errorcluster)  [unwired: 1 in]
                          n150 = local write "error?"(w381) -> ()
                        }
                      }
                    }
                    frame True {
                      n151 = local read "Mode"() -> (w395:u16)
                      n152 = call "compliancevi3subvi.vi"("compliance (A)"=w391, "start"=w386, "compliance (V)"=w390, "total points"=w389, "step"=w385, "Mode"=w395) -> ("total points 2"=w388:u16, "compliance"=w387:dbl)  [unwired: 1 in, 1 out]
                      n153 = call "HP415xA _Config-Sweep-Secondary Sour.vi"("compliance"=w387, "step"=w385, "error in (no error)"=w394, "total points"=w388, "start"=w386, "VISA session"=w393) -> ("error out"=w392:errorcluster)  [unwired: 1 in]
                      n154 = local write "error?"(w392) -> ()
                    }
                  }
                }
              }
            }
            frame True {
              w405 = u16 2 items=["disabled", "Var1", "Var2", "Var1'", "Constant"] ("Function")
              n155 = local read "Mode 2"() -> (w414:u16)
              n156 = local read "Function"() -> (w404:u16)
              n157 = Equal?(x=w404, y=w405) -> (x = y?=w403:bool)
              n158 = local read "error?"() -> (w406:errorcluster)
              n159 = call "compliancesubvi2.vi"("compliance (V)"=w412, "Mode"=w414, "compliance (A)"=w413) -> ("compliance"=w415:dbl)  [unwired: 3 in, 1 out]
              n160 = call "HP415xA _Config-Sweep-Primary Sour.vi"("step (linear only)"=w408, "stop"=w407, "start"=w409, "compliance"=w415, "error in (no error)"=w406, "sweep mode"=w411, "sweep spacing (linear: 0)"=w410, "VISA session"=w399) -> ("error out"=w398:errorcluster)  [unwired: 2 in]
              n161 = case shown="True" w403 {
                tunnel: w402 -> [w421 w464]
                tunnel: w401 -> [w420 w463]
                tunnel: w400 -> [w418 w459]
                tunnel: w399 -> [w423 w469]
                tunnel: w398 -> [w417 w468]
                tunnel: w397 -> [w419 w465]
                tunnel: w396 -> [w416 w461]
                frame False {
                  w425 = u16 2 items=["disabled", "Var1", "Var2", "Var1'", "Constant"] ("Function")
                  n162 = local read "Function 3"() -> (w424:u16)
                  n163 = Equal?(x=w424, y=w425) -> (x = y?=w422:bool)
                  n164 = case shown="True" w422 {
                    tunnel: w423 -> [w431 w457]
                    tunnel: w421 -> [w430 w454]
                    tunnel: w420 -> [w428 w452]
                    tunnel: w419 -> [w429 w453]
                    tunnel: w418 -> [w426 w450]
                    tunnel: w417 -> [w432 w456]
                    tunnel: w416 -> [w427 w448]
                    frame False {
                      w435 = u16 2 items=["disabled", "Var1", "Var2", "Var1'", "Constant"] ("Function")
                      n165 = local read "Function 4"() -> (w434:u16)
                      n166 = Equal?(x=w434, y=w435) -> (x = y?=w433:bool)
                      n167 = case shown="True" w433 {
                        tunnel: w432 -> [w436 w447]
                        tunnel: w431 -> [_ w446]
                        tunnel: w430 -> [_ w443]
                        tunnel: w429 -> [_ w444]
                        tunnel: w428 -> [_ w442]
                        tunnel: w427 -> [_ w438]
                        tunnel: w426 -> [_ w439]
                        frame False {
                          n168 = local write "error?"(w436) -> ()
                        }
                        frame True {
                          n169 = local read "Mode 4"() -> (w441:u16)
                          n170 = call "compliancevi3subvi.vi"("compliance (A)"=w443, "start"=w439, "compliance (V)"=w442, "total points"=w444, "step"=w438, "Mode"=w441) -> ("total points 2"=w440:u16, "compliance"=w437:dbl)  [unwired: 1 in, 1 out]
                          n171 = call "HP415xA _Config-Sweep-Secondary Sour.vi"("compliance"=w437, "step"=w438, "error in (no error)"=w447, "total points"=w440, "start"=w439, "VISA session"=w446) -> ("error out"=w445:errorcluster)  [unwired: 1 in]
                          n172 = local write "error?"(w445) -> ()
                        }
                      }
                    }
                    frame True {
                      n173 = local read "Mode 3"() -> (w458:u16)
                      n174 = call "compliancevi3subvi.vi"("compliance (A)"=w454, "start"=w450, "compliance (V)"=w452, "total points"=w453, "step"=w448, "Mode"=w458) -> ("total points 2"=w451:u16, "compliance"=w449:dbl)  [unwired: 1 in, 1 out]
                      n175 = call "HP415xA _Config-Sweep-Secondary Sour.vi"("compliance"=w449, "step"=w448, "error in (no error)"=w456, "total points"=w451, "start"=w450, "VISA session"=w457) -> ("error out"=w455:errorcluster)  [unwired: 1 in]
                      n176 = local write "error?"(w455) -> ()
                    }
                  }
                }
                frame True {
                  n177 = local read "Mode"() -> (w466:u16)
                  n178 = call "compliancevi3subvi.vi"("compliance (A)"=w464, "start"=w459, "compliance (V)"=w463, "total points"=w465, "step"=w461, "Mode"=w466) -> ("total points 2"=w460:u16, "compliance"=w462:dbl)  [unwired: 1 in, 1 out]
                  n179 = call "HP415xA _Config-Sweep-Secondary Sour.vi"("compliance"=w462, "step"=w461, "error in (no error)"=w468, "total points"=w460, "start"=w459, "VISA session"=w469) -> ("error out"=w467:errorcluster)  [unwired: 1 in]
                  n180 = local write "error?"(w467) -> ()
                }
              }
            }
          }
        }
        frame True {
          w478 = u16 2 items=["disabled", "Var1", "Var2", "Var1'", "Constant"] ("Function 2")
          n181 = local read "error?"() -> (w480:errorcluster)
          n182 = local read "Mode"() -> (w488:u16)
          n183 = local read "Function 2"() -> (w479:u16)
          n184 = call "compliancesubvi2.vi"("compliance (V)"=w487, "Mode"=w488, "compliance (A)"=w486) -> ("compliance"=w489:dbl)  [unwired: 3 in, 1 out]
          n185 = call "HP415xA _Config-Sweep-Primary Sour.vi"("step (linear only)"=w483, "stop"=w482, "start"=w481, "compliance"=w489, "error in (no error)"=w480, "sweep mode"=w484, "sweep spacing (linear: 0)"=w485, "VISA session"=w470) -> ("error out"=w471:errorcluster)  [unwired: 2 in]
          n186 = Equal?(x=w479, y=w478) -> (x = y?=w477:bool)
          n187 = case shown="True" w477 {
            tunnel: w476 -> [w495 w539]
            tunnel: w475 -> [w496 w538]
            tunnel: w474 -> [w493 w535]
            tunnel: w473 -> [w494 w537]
            tunnel: w472 -> [w492 w533]
            tunnel: w471 -> [w491 w542]
            tunnel: w470 -> [w490 w540]
            frame False {
              w499 = u16 2 items=["disabled", "Var1", "Var2", "Var1'", "Constant"] ("Function 2")
              n188 = local read "Function 3"() -> (w498:u16)
              n189 = Equal?(x=w498, y=w499) -> (x = y?=w497:bool)
              n190 = case shown="True" w497 {
                tunnel: w496 -> [w504 w522]
                tunnel: w495 -> [w505 w523]
                tunnel: w494 -> [w502 w528]
                tunnel: w493 -> [w503 w525]
                tunnel: w492 -> [w501 w524]
                tunnel: w491 -> [w506 w531]
                tunnel: w490 -> [w500 w529]
                frame False {
                  w509 = u16 2 items=["disabled", "Var1", "Var2", "Var1'", "Constant"] ("Function 2")
                  n191 = local read "Function 4"() -> (w508:u16)
                  n192 = Equal?(x=w508, y=w509) -> (x = y?=w507:bool)
                  n193 = case shown="True" w507 {
                    tunnel: w506 -> [w510 w521]
                    tunnel: w505 -> [_ w511]
                    tunnel: w504 -> [_ w512]
                    tunnel: w503 -> [_ w513]
                    tunnel: w502 -> [_ w518]
                    tunnel: w501 -> [_ w515]
                    tunnel: w500 -> [_ w519]
                    frame False {
                      n194 = local write "error?"(w510) -> ()
                    }
                    frame True {
                      n195 = local read "Mode 4"() -> (w517:u16)
                      n196 = call "compliancevi3subvi.vi"("compliance (A)"=w511, "start"=w513, "compliance (V)"=w512, "total points"=w518, "step"=w515, "Mode"=w517) -> ("total points 2"=w514:u16, "compliance"=w516:dbl)  [unwired: 1 in, 1 out]
                      n197 = call "HP415xA _Config-Sweep-Secondary Sour.vi"("compliance"=w516, "step"=w515, "error in (no error)"=w521, "total points"=w514, "start"=w513, "VISA session"=w519) -> ("error out"=w520:errorcluster)  [unwired: 1 in]
                      n198 = local write "error?"(w520) -> ()
                    }
                  }
                }
                frame True {
                  n199 = local read "Mode 3"() -> (w532:u16)
                  n200 = call "compliancevi3subvi.vi"("compliance (A)"=w523, "start"=w525, "compliance (V)"=w522, "total points"=w528, "step"=w524, "Mode"=w532) -> ("total points 2"=w527:u16, "compliance"=w526:dbl)  [unwired: 1 in, 1 out]
                  n201 = call "HP415xA _Config-Sweep-Secondary Sour.vi"("compliance"=w526, "step"=w524, "error in (no error)"=w531, "total points"=w527, "start"=w525, "VISA session"=w529) -> ("error out"=w530:errorcluster)  [unwired: 1 in]
                  n202 = local write "error?"(w530) -> ()
                }
              }
            }
            frame True {
              n203 = local read "Mode 2"() -> (w543:u16)
              n204 = call "compliancevi3subvi.vi"("compliance (A)"=w539, "start"=w535, "compliance (V)"=w538, "total points"=w537, "step"=w533, "Mode"=w543) -> ("total points 2"=w536:u16, "compliance"=w534:dbl)  [unwired: 1 in, 1 out]
              n205 = call "HP415xA _Config-Sweep-Secondary Sour.vi"("compliance"=w534, "step"=w533, "error in (no error)"=w542, "total points"=w536, "start"=w535, "VISA session"=w540) -> ("error out"=w541:errorcluster)  [unwired: 1 in]
              n206 = local write "error?"(w541) -> ()
            }
          }
        }
      }
    }
    frame #4 {
      # "This step sets the integration time."
      n207 = local read "VISA session"() -> (w544:refnum<visa-resource-name>)
      n208 = local read "error?"() -> (w548:errorcluster)
      n209 = call "HP415xA _Config-Meas-Timing.vi"("error in (no error)"=w548, "wait time parameter"="wait time parameter", "integration time"="integration time", "VISA session"=w544) -> ("error out"=w547:errorcluster)  [unwired: 2 in]
      n210 = local write "error?"(w547) -> ()
    }
    frame #5 {
      w587 = u32 1 items=["stop  ", "single  ", "single-append  ", "stress start  ", "continuous  ", "standby on  ", "standby off  ", "zero  "] ("function (stop:0)")
      w591 = u16 2 items=["disabled", "Var1", "Var2", "Var1'", "Constant"] ("Function")
      w596 = u16 1 items=["disabled", "Var1", "Var2", "Var1'", "Constant"] ("Function")
      n211 = local read "Function"() -> (w598:u16)
      n212 = local read "Function"() -> (w590:u16)
      n213 = Equal?(x=w598, y=w596) -> (x = y?=w597:bool)
      n214 = Equal?(x=w590, y=w591) -> (x = y?=w589:bool)
      n215 = case shown="False" w597 {
        tunnel: [w885 w900] -> w592
        tunnel: [w886 w899] -> _
        tunnel: w596 -> [w883 _]
        frame False {
          n216 = local read "Function 2"() -> (w887:u16)
          n217 = Equal?(x=w887, y=w883) -> (x = y?=w884:bool)
          n218 = case shown="False" w884 {
            tunnel: [w888 w898] -> w886
            tunnel: [w889 w897] -> w885
            tunnel: w883 -> [w892 _]
            frame False {
              n219 = local read "Function 3"() -> (w891:u16)
              n220 = Equal?(x=w891, y=w892) -> (x = y?=w890:bool)
              n221 = case shown="True" w890 {
                tunnel: [w894 w896] -> w889
                tunnel: [w893 w895] -> w888
                frame False {
                  n222 = local read "Vname 4"() -> (w894:string)
                  n223 = local read "Iname 4"() -> (w893:string)
                }
                frame True {
                  n224 = local read "Vname 3"() -> (w896:string)
                  n225 = local read "Iname 3"() -> (w895:string)
                }
              }
            }
            frame True {
              n226 = local read "Iname 2"() -> (w898:string)
              n227 = local read "Vname 2"() -> (w897:string)
            }
          }
        }
        frame True {
          n228 = local read "Vname"() -> (w900:string)
          n229 = local read "Iname"() -> (w899:string)
        }
      }
      n230 = case shown="False" w589 {
        tunnel: [w827 w880] -> w552
        tunnel: [w826 TRUE ("x = y?")] -> w569
        frame False {
          w830 = u16 2 items=["disabled", "Var1", "Var2", "Var1'", "Constant"] ("Function")
          n231 = local read "Function 2"() -> (w829:u16)
          n232 = Equal?(x=w829, y=w830) -> (x = y?=w828:bool)
          n233 = case shown="True" w828 {
            tunnel: [w832 w870] -> w827
            tunnel: [w831 TRUE ("x = y?")] -> w826
            frame False {
              w835 = u16 2 items=["disabled", "Var1", "Var2", "Var1'", "Constant"] ("Function")
              n234 = local read "Function 3"() -> (w834:u16)
              n235 = Equal?(x=w834, y=w835) -> (x = y?=w833:bool)
              n236 = case shown="True" w833 {
                tunnel: [w840 w860] -> w832
                tunnel: [w836 TRUE ("x = y?")] -> w831
                frame False {
                  w839 = u16 2 items=["disabled", "Var1", "Var2", "Var1'", "Constant"] ("Function")
                  n237 = local read "Function 4"() -> (w838:u16)
                  n238 = Equal?(x=w838, y=w839) -> (x = y?=w837:bool)
                  n239 = case shown="True" w837 {
                    tunnel: ["0" ("Vname 4") w850] -> w840
                    tunnel: [FALSE ("x = y?") TRUE ("x = y?")] -> w836
                    frame False {
                    }
                    frame True {
                      w844 = u16 2 items=["V", "I", "VPulse", "IPulse", "Common"] ("Mode 2")
                      w847 = u16 0 items=["V", "I", "VPulse", "IPulse", "Common"] ("Mode 2")
                      n240 = local read "Mode 4"() -> (w846:u16)
                      n241 = Equal?(x=w847, y=w846) -> (x = y?=w848:bool)
                      n242 = Equal?(x=w846, y=w844) -> (x = y?=w845:bool)
                      n243 = Or(x=w848, y=w845) -> (x .or. y?=w843:bool)
                      n244 = case shown="False" w843 {
                        tunnel: [w851 w852] -> w850
                        frame False {
                          n245 = local read "Iname 4"() -> (w851:string)
                        }
                        frame True {
                          n246 = local read "Vname 4"() -> (w852:string)
                        }
                      }
                    }
                  }
                }
                frame True {
                  w856 = u16 2 items=["V", "I", "VPulse", "IPulse", "Common"] ("Mode 2")
                  w855 = u16 0 items=["V", "I", "VPulse", "IPulse", "Common"] ("Mode 2")
                  n247 = local read "Mode 3"() -> (w854:u16)
                  n248 = Equal?(x=w855, y=w854) -> (x = y?=w858:bool)
                  n249 = Equal?(x=w854, y=w856) -> (x = y?=w857:bool)
                  n250 = Or(x=w858, y=w857) -> (x .or. y?=w853:bool)
                  n251 = case shown="False" w853 {
                    tunnel: [w861 w862] -> w860
                    frame False {
                      n252 = local read "Iname 3"() -> (w861:string)
                    }
                    frame True {
                      n253 = local read "Vname 3"() -> (w862:string)
                    }
                  }
                }
              }
            }
            frame True {
              w864 = u16 2 items=["V", "I", "VPulse", "IPulse", "Common"] ("Mode 2")
              w865 = u16 0 items=["V", "I", "VPulse", "IPulse", "Common"] ("Mode 2")
              n254 = local read "Mode 2"() -> (w866:u16)
              n255 = Equal?(x=w865, y=w866) -> (x = y?=w868:bool)
              n256 = Equal?(x=w866, y=w864) -> (x = y?=w867:bool)
              n257 = Or(x=w868, y=w867) -> (x .or. y?=w863:bool)
              n258 = case shown="True" w863 {
                tunnel: [w871 w872] -> w870
                frame False {
                  n259 = local read "Iname 2"() -> (w871:string)
                }
                frame True {
                  n260 = local read "Vname 2"() -> (w872:string)
                }
              }
            }
          }
        }
        frame True {
          w877 = u16 2 items=["V", "I", "VPulse", "IPulse", "Common"] ("Mode")
          w878 = u16 0 items=["V", "I", "VPulse", "IPulse", "Common"] ("Mode")
          n261 = local read "Mode"() -> (w876:u16)
          n262 = Equal?(x=w876, y=w878) -> (x = y?=w875:bool)
          n263 = Equal?(x=w876, y=w877) -> (x = y?=w874:bool)
          n264 = Or(x=w875, y=w874) -> (x .or. y?=w873:bool)
          n265 = case shown="True" w873 {
            tunnel: [w881 w882] -> w880
            frame False {
              n266 = local read "Iname"() -> (w881:string)
            }
            frame True {
              n267 = local read "Vname"() -> (w882:string)
            }
          }
        }
      }
      n268 = local read "error?"() -> (w579:errorcluster)
      n269 = Unbundle("Y2 axis settings") -> ("Y2 axis on/off"=w572:bool, "MINIMUM"=w584:ext, "MAXIMUM"=w583:ext, "Variable name"=w575:string, "LIN or LOG axis"=w582:string)
      n270 = local read "Var2 step settings"() -> (w594:T6)
      n271 = local read "Var1 sweep settings"() -> (w595:T7)
      n272 = local read "VISA session"() -> (w564:refnum<visa-resource-name>)
      n273 = call "Y1subvi.vi"("MAXIMUM"="MAXIMUM", "Variable name"="Y1 axis", "error in (no error)"=w579, "MINIMUM"="MINIMUM", "LIN or LOG axis"="LIN", "VISA resource name"=w564) -> ("error out"=w580:errorcluster)
      n274 = case shown="False" w572 {
        tunnel: w580 -> [w818 w825]
        tunnel: w564 -> [_ w824]
        tunnel: w584 -> [_ w823]
        tunnel: w583 -> [_ w822]
        tunnel: w575 -> [_ w821]
        tunnel: w582 -> [_ w820]
        tunnel: [w818 w819] -> w581
        frame False {
        }
        frame True {
          n275 = call "Y2subvi.vi"("MAXIMUM"=w822, "Variable name"=w821, "error in (no error)"=w825, "MINIMUM"=w823, "LIN or LOG axis"=w820, "VISA resource name"=w824) -> ("error out"=w819:errorcluster)
        }
      }
      n276 = Unbundle(w594) -> ("total points"=w593:u16)  [unwired: 4 out]
      n277 = Decrement(x=w593) -> (x-1=w555:u16)
      n278 = Unbundle(w595) -> ("start"=w563:dbl)  [unwired: 6 out]
      n279 = call "HP415xA Op-Start-Stop.vi"("error in (no error)"=w581, "function (stop:0)"=w587, "wait until finish"=TRUE, "VISA session"=w564) -> ("error out"=w586:errorcluster)  [unwired: 6 in, 1 out]
      n280 = call "HP415xA Op-Download Trace.vi"("error in (no error)"=w586, "trace (variable) name"=w592, "VISA session"=w564) -> ("error out"=w601:errorcluster, "trace"=w570:dbl[])
      n281 = call "HP415xA Op-Download Trace.vi"("error in (no error)"=w601, "trace (variable) name"="Y1 axis", "VISA session"=w564) -> ("error out"=w576:errorcluster, "trace"=w565:dbl[])
      n282 = case shown="False" w572 {
        tunnel: w576 -> [w802 w811]
        tunnel: w564 -> [_ w810]
        tunnel: w575 -> [_ w809]
        tunnel: [w802 w808] -> w566
        tunnel: w570 -> [w800 w807]
        tunnel: w565 -> [w801 w806]
        tunnel: [w799 w805] -> w551
        tunnel: [dbl[] [] ("trace") w804] -> w571
        tunnel: [cluster{"trace":dbl[], "trace":dbl[]} {"trace"=[], "trace"=[]} w803] -> w549
        frame False {
          n283 = Bundle("trace"=w800, "trace"=w801) -> (w799:cluster{"trace":dbl[], "trace":dbl[]})  [unwired: 1 in]
        }
        frame True {
          n284 = call "HP415xA Op-Download Trace.vi"("error in (no error)"=w811, "trace (variable) name"=w809, "VISA session"=w810) -> ("error out"=w808:errorcluster, "trace"=w804:dbl[])
          n285 = stacked-sequence {
            tunnel: w804 -> [_ w817]
            tunnel: w807 -> [w814 w816]
            tunnel: w806 -> [w813 _]
            tunnel: [w812 _] -> w805
            tunnel: [_ w815] -> w803
            frame #0 {
              n286 = Bundle("trace"=w814, "trace"=w813) -> (w812:cluster{"trace":dbl[], "trace":dbl[]})  [unwired: 1 in]
            }
            frame #1 {
              n287 = Bundle("trace"=w816, "trace"=w817) -> (w815:cluster{"trace":dbl[], "trace":dbl[]})  [unwired: 1 in]
              "Gate Current Plot" <- w815
            }
          }
        }
      }
      "graphic display" <- w551
      n288 = Build Array(w549) -> (w550:cluster{"trace":dbl[], "trace":dbl[]}[])
      n289 = case shown="True" w569 {
        tunnel: w563 -> [_ w723]
        tunnel: w565 -> [w606 w722]
        tunnel: w570 -> [w607 w721]
        tunnel: w555 -> [_ w720]
        tunnel: w564 -> [_ w716]
        tunnel: w566 -> [_ w715]
        tunnel: [w608 w714] -> w568
        tunnel: w552 -> [_ w713]
        tunnel: w552 -> [_ w706]
        tunnel: [dbl[] [] ("trace") w712] -> w567
        tunnel: w562 -> [_ w709]
        tunnel: w561 -> [_ w708]
        tunnel: w560 -> [_ w685]
        tunnel: [_ w617] -> w559
        tunnel: [_ w612] -> w558
        tunnel: w557 -> [_ w687]
        tunnel: w556 -> [_ w686]
        tunnel: w555 -> [_ _]
        tunnel: w554 -> [_ _]
        tunnel: w553 -> [_ w668]
        tunnel: w550 -> [_ w609]
        frame False {
          n290 = Build Array(w607, w606) -> (w603:dbl[][])
          n291 = local read "error? 2"() -> (w608:errorcluster)
          n292 = call-poly <vilib>:"Write To Spreadsheet File.vi"("transpose? (no:F)"=TRUE ("append to file? (new file:F)"), "format (%.3f)"="%.5e", "2D data"=w603) -> ()  [unwired: 5 in, 1 out]
        }
        frame True {
          (unwired) "\r"
          w679 = "\r"
          # "Find Smallest Vd Value"
          # "Picks linear Id based on Smallest Vd"
          # "Dielectric"
          # "Data Values"
          # "Headers"
          n293 = call "HP415xA Op-Download Trace.vi"("error in (no error)"=w715, "trace (variable) name"=w713, "VISA session"=w716) -> ("error out"=w714:errorcluster, "trace"=w712:dbl[])
          n294 = Initialize Array("") -> (w689:string[])  [unwired: 1 in]
          n295 = for {
            N: w720 -> [w724]
            shift-right: [w741] -> w617
            shift-left: w721 -> [w737]
            tunnel: w723 -> [w743]
            tunnel: [w742] -> _ mode=indexing
            shift-right: [w738] -> w612
            shift-left: w722 -> [w740]
            tunnel: [w739] -> w661 mode=indexing
            shift-right: [w734] -> w703
            shift-left: w712 -> [w736]
            tunnel: w706 -> [_]
            tunnel: [w728] -> w663 mode=indexing
            shift-right: [w727] -> w693
            shift-left: w689 -> [w726]
            tunnel: [w724] -> _ mode=indexing
            # "Cuts data at each new loop"
            # "Id Data"
            # "Vd Data"
            # "Vg Data"
            n296 = Search 1D Array(1D array=w737, element=w743, start index (0)=1) -> (index of element=w735:i32)
            n297 = Split 1D Array(array=w736, index=w735) -> (first subarray=w732:dbl[], second subarray=w734:dbl[])
            n298 = Split 1D Array(array=w737, index=w735) -> (first subarray=w742:dbl[], second subarray=w741:dbl[])
            n299 = Split 1D Array(array=w740, index=w735) -> (first subarray=w739:dbl[], second subarray=w738:dbl[])
            n300 = Array Size(array=w732) -> (size(s)=w731:i32)
            n301 = Decrement(x=w731) -> (x-1=w730:i32)
            n302 = Array Subset(array=w732, index=w730) -> (w733:dbl[])  [unwired: 1 in]
            n303 = Number To Exponential String(number=w733) -> (E-format string=w729:string[])  [unwired: 3 in]
            n304 = Build Array (concatenate)("Id", w726) -> (w727:string[])
            n305 = Concatenate Strings(w729) -> (w728:string)
          }
          n306 = local read "Temp (K)"() -> (w640:dbl)
          n307 = Fract/Exp String To Number(string=w686) -> (number=w666:dbl)  [unwired: 3 in, 1 out]
          n308 = Fract/Exp String To Number(string=w687) -> (number=w667:dbl)  [unwired: 3 in, 1 out]
          n309 = local read "Temp (K)"() -> (w657:dbl)
          n310 = local read "NumPts"() -> (w665:dbl)
          n311 = local read "NumPts"() -> (w658:dbl)
          n312 = Fract/Exp String To Number(string=w668) -> (number=w659:dbl)  [unwired: 3 in, 1 out]
          n313 = Array Size(array=w703) -> (size(s)=w704:i32)
          n314 = call "STS Calculator.vi"("NumPts"=w658, "Saturation Id"=w612, "Vg Column"=w617) -> ("Sub Threshold Swing"=w651:dbl)  [unwired: 5 in, 3 out]
          n315 = call "Mobility-Vt Calculator_Saturation_12_09_10a_JW.vi"("Vg Column"=w617, "Sat Id Column"=w612, "NumPts"=w658, "Length"=w666, "Width"=w667, "Dielectric Thickness"=w659) -> ("Check Cluster"=w647:T8, "Mobility-Sat"=w656:dbl, "VT-Sat"=w652:dbl, "Off I-Sat"=w653:dbl, "On/Off I-Sat"=w654:dbl)  [unwired: 1 in, 4 out]
          n316 = local write "Check Cluster"(w647) -> ()
          n317 = Decrement(x=w704) -> (x-1=w702:i32)
          n318 = call "Trap Density_VT.vi"("VT"=w652, "Dielectric"=w659) -> ("Trap Density-VT"=w650:dbl)
          n319 = call "Trap Density_STS.vi"("Temp (T) [K]"=w657, "S.T.S. (S)"=w651, "Dielectric"=w659) -> ("Trap Density (N)"=w649:dbl)  [unwired: 8 in]
          n320 = Array Subset(array=w703, index=w702) -> (w701:dbl[])  [unwired: 1 in]
          n321 = Number To Exponential String(number=w701) -> (E-format string=w697:string[])  [unwired: 3 in]
          n322 = Build Array("Sample Temp (K):", "", "Mobility-Sat (cm^2/Vs):", "Mobility-Lin (cm^2/Vs):", "On/Off I-Sat:", "Off I-Sat (A):", "Vt-Sat (V):", "STS-Sat (V/decade):", "Trap Density-VT (Traps/Vcm^2):", "Trap Density-STS (Traps/Vcm^2):") -> (w683:string[])
          n323 = Build Array (concatenate)(w617, w661, w612) -> (w719:dbl[][])
          n324 = Concatenate Strings(w697) -> (w662:string)
          n325 = Build Array (concatenate)(w663, w662) -> (w660:string[])
          n326 = Fract/Exp String To Number(string=w660) -> (number=w645:dbl[])  [unwired: 3 in, 1 out]
          n327 = Build Array (concatenate)(w661, w612) -> (w643:dbl[][])
          n328 = Build Array("Vg", "Id") -> (w694:string[])
          n329 = Absolute Value(x=w645) -> (abs(x)=w646:dbl[])
          n330 = Insert Into Array(array=w694, index=2, new element=w693) -> (w692:string[])
          n331 = Array Max & Min(array=w646) -> (min index (indices)=w642:i32)  [unwired: 3 out]
          n332 = Index Array(array=w645, index=w642) -> (element=w644:dbl)
          n333 = Build Array (concatenate)("Vd=", w663, w662) -> (w700:string[])
          n334 = Transpose 2D Array(2D array=w719) -> (transposed array=w717:dbl[][])
          n335 = Index Array(array=w643, index (row)=w642) -> (element=w614:dbl[])  [unwired: 1 in]
          n336 = call "Mobility-Vt Calculator_Linear.vi"("Vg Column"=w617, "Vd"=w644, "Lin Id Column"=w614, "NumPts"=w665, "Length"=w666, "Width"=w667, "Dielectric Thickness"=w659) -> ("Mobility-Lin"=w655:dbl)  [unwired: 2 in, 6 out]
          n337 = Build Array(w640, w656, w655, w654, w653, w652, w651, w650, w649) -> (w682:dbl[])
          n338 = Number To Exponential String(number=w682) -> (E-format string=w639:string[])  [unwired: 3 in]
          n339 = Bundle("Mobility-Sat"=w656, "Mobility-Lin"=w655, "On/Off I-Sat"=w654, "Off I-Sat"=w653, "VT-Sat"=w652, "Sub Threshold Swing"=w651, "Trap Density-VT"=w650, "Trap Density (N)"=w649) -> (w648:T9)  [unwired: 1 in]
          n340 = local write "Output"(w648) -> ()
          n341 = Insert Into Array(array=w639, index=1, new element="") -> (w636:string[])
          n342 = Build Array(w683, w636) -> (w635:string[][])
          n343 = Transpose 2D Array(2D array=w635) -> (transposed array=w634:string[][])
          n344 = Array To Spreadsheet String(array=w700, 3:"%s") -> (spreadsheet string=w705:string)  [unwired: 1 in]
          n345 = Array To Spreadsheet String(array=w692, 3:"%s") -> (spreadsheet string=w698:string)  [unwired: 1 in]
          n346 = Array To Spreadsheet String(array=w634, 3:"%s") -> (spreadsheet string=w680:string)  [unwired: 1 in]
          n347 = Array To Spreadsheet String(array=w717, 3:"%.5e" ("format string")) -> (spreadsheet string=w707:string)  [unwired: 1 in]
          n348 = Concatenate Strings(w709, w679, w708, w679, w685, w680, w679, w705, w698, w707, "\r") -> (w711:string)
          n349 = Absolute Value(x=w614) -> (abs(x)=w619:dbl[])
          n350 = Absolute Value(x=w612) -> (abs(x)=w616:dbl[])
          n351 = Absolute Value(x=w614) -> (abs(x)=w613:dbl[])
          n352 = Absolute Value(x=w612) -> (abs(x)=w611:dbl[])
          n353 = Square Root(x=w619) -> (sqrt(x)=w618:dbl[])
          n354 = Square Root(x=w616) -> (sqrt(x)=w615:dbl[])
          n355 = local read "Input Path"() -> (w669:path)
          n356 = Bundle("trace"=w617, w613) -> (w622:cluster{"trace":dbl[], dbl[]})  [unwired: 1 in]
          n357 = Bundle("trace"=w617, w611) -> (w625:cluster{"trace":dbl[], dbl[]})  [unwired: 1 in]
          n358 = Bundle("trace"=w617, w618) -> (w621:cluster{"trace":dbl[], dbl[]})  [unwired: 1 in]
          n359 = Bundle("trace"=w617, w615) -> (w626:cluster{"trace":dbl[], dbl[]})  [unwired: 1 in]
          n360 = Bundle("trace"=w617, w614) -> (w628:cluster{"trace":dbl[], dbl[]})  [unwired: 1 in]
          n361 = Bundle("trace"=w617, "trace"=w612) -> (w630:cluster{"trace":dbl[], "trace":dbl[]})  [unwired: 1 in]
          n362 = Build Array(w621) -> (w620:cluster{"trace":dbl[], dbl[]}[])
          n363 = Build Array(w622) -> (w610:cluster{"trace":dbl[], dbl[]}[])
          n364 = Build Array(w626) -> (w623:cluster{"trace":dbl[], dbl[]}[])
          n365 = Build Array(w625) -> (w624:cluster{"trace":dbl[], dbl[]}[])
          n366 = Build Array(w628) -> (w627:cluster{"trace":dbl[], dbl[]}[])
          n367 = Build Array(w630) -> (w629:cluster{"trace":dbl[], "trace":dbl[]}[])
          n368 = call <vilib>:"Write Characters To File.vi"("append to file? (new file:F)"=TRUE, "character string"=w711, "file path (dialog if empty)"=w669) -> ("new file path (Not A Path if cancelled)"=w677:path)  [unwired: 2 in]
          n369 = local read "Graph Cluster"() -> (w632:T1)
          n370 = local write "Output Path"(w677) -> ()
          n371 = Bundle By Name(cluster=w632, "Linear Sqrt"=w620, "Linear Log"=w610, "Linear Raw"=w627, "Saturation Sqrt"=w623, "Saturation Log"=w624, "Saturation Raw"=w629, "Gate Current"=w609) -> (w631:T1)
          n372 = local write "Graph Cluster"(w631) -> ()
        }
      }
      n373 = case shown="True" w572 {
        tunnel: w555 -> [_ w750]
        tunnel: w569 -> [_ w751]
        tunnel: w570 -> [_ w749]
        tunnel: w563 -> [_ w748]
        tunnel: w571 -> [_ w747]
        tunnel: w567 -> [_ w746]
        tunnel: w552 -> [_ w745]
        frame False {
        }
        frame True {
          n374 = case shown="True" w751 {
            tunnel: w750 -> [_ w767]
            tunnel: w749 -> [w755 w782]
            tunnel: w748 -> [_ w781]
            tunnel: w747 -> [w756 w780]
            tunnel: w746 -> [_ w779]
            tunnel: w745 -> [_ w762]
            frame False {
              n375 = Build Array(w755, w756) -> (w754:dbl[][])
              n376 = call-poly <vilib>:"Write To Spreadsheet File.vi"("transpose? (no:F)"=TRUE, "format (%.3f)"="%.5e", "2D data"=w754) -> ()  [unwired: 5 in, 1 out]
            }
            frame True {
              n377 = for {
                N: w767 -> [_]
                shift-right: [w793] -> w778
                shift-left: w782 -> [w794]
                tunnel: w781 -> [w796]
                tunnel: [w792] -> _ mode=indexing
                shift-right: [w789] -> w776
                shift-left: w780 -> [w791]
                tunnel: [w790] -> w777 mode=indexing
                shift-right: [w786] -> w771
                shift-left: w779 -> [w787]
                tunnel: [w783] -> w768 mode=indexing
                n378 = Search 1D Array(1D array=w794, element=w796, start index (0)=1) -> (index of element=w788:i32)
                n379 = Split 1D Array(array=w794, index=w788) -> (first subarray=w792:dbl[], second subarray=w793:dbl[])
                n380 = Split 1D Array(array=w791, index=w788) -> (first subarray=w790:dbl[], second subarray=w789:dbl[])
                n381 = Split 1D Array(array=w787, index=w788) -> (first subarray=w784:dbl[], second subarray=w786:dbl[])
                n382 = Index Array(array=w784, index=1) -> (element=w783:dbl)
              }
              n383 = Build Array (concatenate)(w778, w777, w776) -> (w775:dbl[][])
              n384 = Index Array(array=w771, index=1) -> (element=w769:dbl)
              n385 = Transpose 2D Array(2D array=w775) -> (transposed array=w774:dbl[][])
              n386 = Insert Into Array(array=w768, index=w767, new element=w769) -> (w766:dbl[])
              n387 = Array To Spreadsheet String(delimiter (Tab)=",", array=w766, 3:"%.5e" ("format string")) -> (spreadsheet string=w760:string)
              n388 = Array To Spreadsheet String(delimiter (Tab)=",", array=w774, 3:"%.5e" ("format string")) -> (spreadsheet string=w758:string)
              n389 = Concatenate Strings(w762, "," ("string")) -> (w761:string)
              n390 = Concatenate Strings(w761, w760) -> (w759:string)
              n391 = Concatenate Strings(w759, w758) -> (w757:string)
              n392 = call <vilib>:"Write Characters To File.vi"("character string"=w757) -> ()  [unwired: 4 in, 1 out]
            }
          }
        }
      }
      n393 = call "HP415xA Sys-Error Query.vi"("VISA session"=w564, "error in (no error)"=w568) -> ("error out"=w599:errorcluster)  [unwired: 2 in, 1 out]
      n394 = call "HP415xA  Close.vi"("error in (no error)"=w599, "VISA session"=w564) -> ("error out"=w600:errorcluster)
      n395 = local write "error?"(w600) -> ()
    }
  }
